vi "Q14070-Z060B手动版.vi"() -> ()   [LabVIEW 2013]
uses:
  <vilib>/Utility/file.llb/Read From Spreadsheet File (string).vi
  <vilib>/express/express arith-compare/Formula/XNode/ExpressFormulaBlockNode.xnode
  PCI8622_32.dll
  <vilib>/printing/EasyPrintingControls.llb/contents.ctl
  <vilib>/Utility/NIReport.llb/NI_ReportGenerationCore.lvlib
  <vilib>/printing/EasyPrintingControls.llb/report_type.ctl
  <vilib>/Utility/NIReport.llb/NI_report.lvclass
  <vilib>/printing/EasyPrinting.llb/Easy Print VI Panel or Documentation (path).vi
panel:
  out "界面启动":bool
  out "间隙扭矩扳手信号":bool
  out "齿条右极限":dbl
  out "齿条左极限":dbl
  out "左轴向力数组大小":i32
  in  "电动缸快速":dbl=10.0
  in  "电动缸慢速":dbl=1.0
  out "最大轴向力标准(N)":dbl=200.0 caption="L+Lmax(mm)" format="%#.3f"
  out "循环退出":bool
  in  "?":bool
  in  "密码":string
  in  "?":bool
  in  "?":bool
  in  "截取百分比":dbl=0.05
  in  "半行程":dbl=70.0
  out "PLC":bool
  out "齿条传动比":dbl=200.0 caption="L+Lmax(mm)" format="%#.3f"
  out "右平均轴向力(N)":dbl caption="L+Lmax(mm)" format="%#.3f"
  out "左平均轴向力(N)":dbl caption="最大位移偏离Lmax(mm)" format="%#.3f"
  in  "确定按钮":bool
  out "员工ID":string
  in  "出支线工步号":dbl
  out "报警提示":string
  in  "报警工步号":dbl
  out "急停":bool
  out "DeviceHandle":u32
  in  "轴向力设定次数":dbl=5.0
  in  "最小间隙(mm)":dbl=0.0005 format="%#.3f"
  out "本备料状态H":bool
  out "本测试状态H":bool
  out "本自动状态H":bool
  out "夹头松开":bool
  out "测头右位":bool
  out "测头左位":bool
  in  "测头气缸右移":bool
  in  "测头气缸左移":bool
  in  "轴向力已做次数":dbl
  out "轴向力及全行程间隙合格":bool
  out "轴向力启动":bool
  out "间隙启动":bool
  out "夹头夹紧位":bool
  in  "夹头松开":bool
  in  "夹头夹紧":bool
  out "error out":errorcluster
  out "型号数量":i32
  out "error out 4":errorcluster
  in  "间隙设定调整次数":dbl=5.0
  out "读取产品ID":string
  out "本备料状态":bool
  out "本测试状态":bool
  out "本自动状态":bool
  out "FGCS":string
  out "KSJJ":string
  out "Z060BRFID":string
  out "轴向力Y":dbl[](array[numeric])
  out "轴向力X":dbl[](array[numeric])
  out "间隙X数组":dbl[](array[numeric])
  out "间隙Y数组":dbl[](array[numeric])
  out "error out 3":errorcluster caption="错误输出"
  out "rfid工步号":u32
  out "芯片ID":string="201209190001"
  out "rfid完成":bool
  out "rfid触发":bool
  out "本序已做":bool
  in  "回零完成":bool
  in  "电动缸回零":bool
  in  "单点间隙已调试次数":dbl
  in  "需调整角度(度)":dbl
  in  "转向器中心":dbl
  out "扭矩到达":bool
  out "黄灯":bool
  out "红灯":bool
  out "基准位移":dbl caption="压力传感器" format="%#.4f"
  out "上序不合格":bool
  out "单点间隙合格":bool
  out "上序合格":bool
  out "测头机构电机":u32
  out "复位":bool
  in  "型号选择":u16(ring)=2 items=["J709", "J728", "J706"]
  in  "联线按钮":bool
  in  "工步号":u32
  in  "产品ID":string="201209190001"
  out "间隙位移(mm)":dbl=-4.6787895475327215 caption="压力传感器" format="%#.3f"
  out "齿条推拉力(N)":dbl format="%#.2f"
  out "齿条扭矩(Nm)":dbl format="%#.2f"
  out "通讯状态":bool
  out "员工姓名":string
  out "工步提示":string
  out "ADODB._Connection Out 2":refnum<k7>
  out "旋转齿条电机":u32
  out "电动缸电机":u32
  in  "停止":bool
  in  "参数加载":bool
  in  "选项卡控件":T1(tab)
  out "180°外全行程间隙标准(mm)":dbl=0.1 format="%#.3f"
  out "扭动曲线":cluster{"Y":dbl[], "Y":dbl[]}[](graph) caption="压球涨堵头1"
  out "中间位置间隙":dbl caption="间隙值L(mm)" format="%#.3f"
  in  "中间位置最大间隙标准(mm)":dbl=0.07 format="%#.3f"
  out "右180°外全行程间隙":dbl caption="正向最大间隙L1(mm)" format="%#.3f"
  out "左180°外全行程间隙":dbl caption="正向最大间隙L1(mm)" format="%#.3f"
  out "右180°内全行程间隙":dbl caption="正向最大间隙L1(mm)" format="%#.3f"
  out "左180°内全行程间隙":dbl caption="正向最大间隙L1(mm)" format="%#.3f"
  out "180°内全行程间隙标准(mm)":dbl=0.07 format="%#.3f"
  in  "找帽OK":bool
  out "左全行程间隙":dbl caption="正向最大间隙L1(mm)" format="%#.3f"
  out "右全行程间隙":dbl caption="正向最大间隙L1(mm)" format="%#.3f"
  out "总圈数最大值":dbl
  out "总圈数标准":dbl
  out "总行程最大值":dbl
  out "总行程标准(mm)":dbl
  out "力波动标准(N)":dbl=60.0 caption="L+Lmax(mm)" format="%#.3f"
  out "轴向力标准(N)":dbl=100.0 caption="L+Lmax(mm)" format="%#.3f"
  out "右轴向力波动(N)":dbl caption="L+Lmax(mm)" format="%_4g"
  out "右最大轴向力(N)":dbl caption="L+Lmax(mm)" format="%_4g"
  out "左轴向力波动(N)":dbl caption="最大位移偏离Lmax(mm)" format="%_4g"
  out "左最大轴向力(N)":dbl caption="最大位移偏离Lmax(mm)" format="%_4g"
  out "行程跳动曲线":cluster{"Y":dbl[], "Y":dbl[]}[](graph) caption="压球涨堵头1"
  out "平均轴向力标准(N) max":dbl=200.0 caption="L+Lmax(mm)" format="%#.3f"
  out "总行程":dbl format="%_4g"
  out "总圈数":dbl format="%_4g"
  in  "不合格品":bool
  in  "齿条右极限":dbl=-70.0 caption="压力传感器" format="%#.2f"
  in  "齿条左极限":dbl=-262.0 caption="压力传感器" format="%#.2f"
  in  "齿条移动速度":dbl=5.0 caption="压力传感器" format="%#.2f"
  in  "旋转齿条轴找帽转速":dbl=5.0 caption="压力传感器" format="%#.2f"
  in  "测量点扭矩":dbl=4.0 caption="压力传感器" format="%#.2f"
  in  "旋转齿条轴测量转速":dbl caption="压力传感器" format="%#.2f"
  in  "测头机构轴后退位":dbl=30.0 caption="压力传感器" format="%#.2f"
  in  "测头机构轴待检位":dbl caption="压力传感器" format="%#.2f"
  in  "测头机构轴检测位":dbl caption="压力传感器" format="%#.2f"
  in  "测头机构轴移动速度":dbl caption="压力传感器" format="%#.2f"
  in  "机械间隙值":dbl=3.5
  in  "阻挡":bool
  in  "放行":bool
  in  "夹头松开":bool
  in  "夹头夹紧":bool
  in  "测头气缸右移":bool
  in  "测头气缸左移":bool
  in  "支线下降":bool
  in  "支线顶升":bool
  in  "出支线":bool
  in  "进支线":bool
  in  "主线下降":bool
  in  "主线顶升":bool
  in  "下阻挡器放行":bool
  in  "上阻挡器放行":bool
  in  "测头机构轴使能":bool
  in  "测头机构轴后退":bool
  in  "测头机构轴前进":bool
  in  "电动缸速度(mm/s)":dbl=10.0 format="%#.3f"
  out "电动缸位置(mm)":dbl format="%#.3f"
  in  "旋转齿条轴速度(°/s)":dbl=10.0 format="%#.3f"
  out "旋转齿条轴位置(°)":dbl format="%#.3f"
  in  "测头机构轴速度(mm/s)":dbl=10.0 format="%#.3f"
  out "测头机构轴位置(mm)":dbl format="%#.3f"
  in  "旋转齿条轴右转":bool
  in  "旋转齿条轴左转":bool
  in  "旋转齿条轴使能":bool
  in  "电动缸后退":bool
  in  "电动缸使能":bool
  in  "电动缸前进":bool
  in  "齿条扭矩比例偏移":dbl=1.0 format="%#.2f"
  in  "齿条扭矩零点偏移":dbl format="%#.2f"
  in  "齿条推拉力比例偏移":dbl=1.0 format="%#.2f"
  in  "齿条推拉力零点偏移":dbl format="%#.2f"
  in  "间隙位移比例偏移":dbl=1.0 format="%#.2f"
  in  "间隙位移零点偏移":dbl format="%#.2f"
  in  "传感器参数保存":bool
  in  "参数修改":bool
  in  "参数查询":bool
  in  "参数浏览表":string[][](table)
  # "芜湖机械转向器装配线"
  # "间隙及轴向力检测"
  # "湖北唯思凌科装备制造有限公司 设计开发 (C)2015"
  # "Q14070机械转向器装配线"
  # "≤"
  # "间隙测量结果"
  # "间隙测量判定值"
  # "≤"
  # "≤"
  # "≤"
  # "轴向力测量结果"
  # "轴向力测量标准"
  # "≥"
  # "≤"
  # "≥"
  # "≤"
  # "≤"
  # "≥"
  # "不得大于20NM"
  # "传感器校验区"
  # "关于传感器校验：\n1、传感器校验需要由具备资质的单位或部门进行校验。\n2、具备权限的用户才能够修改传感器校验参数和试验参数。\n3、修改校验参数方法：先将比例偏移置为1，修改零点偏移，使零点值与校验的传感器一致；然后根据增幅调整比例偏移。"
  # "注意：\n具备权限的用户才能够修改传感器校验参数和试验参数！"
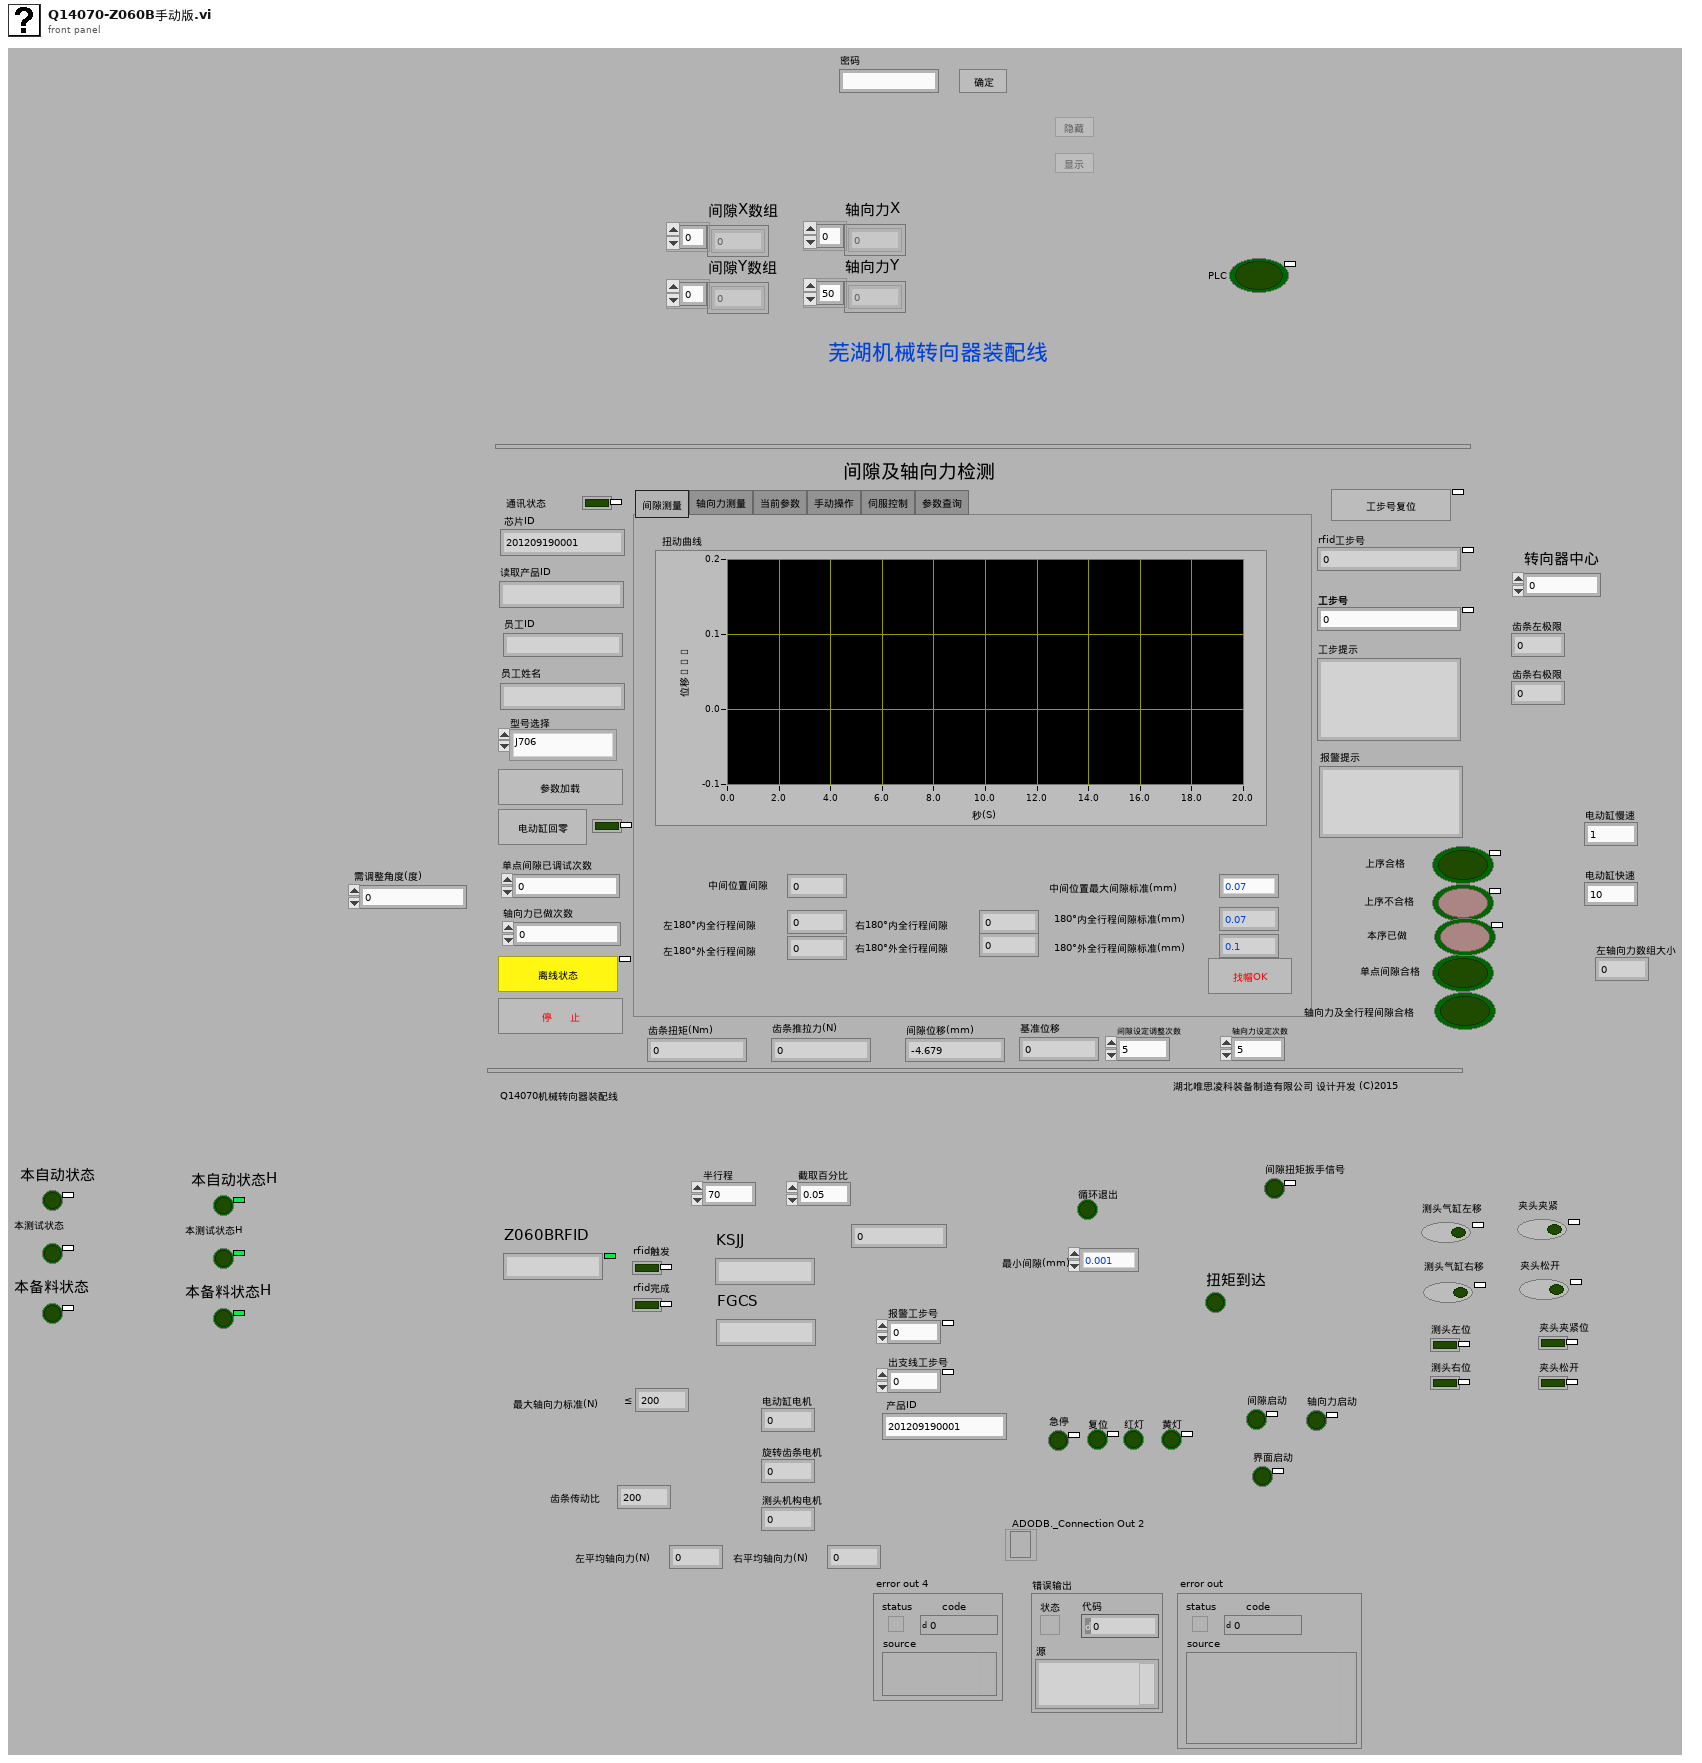
[diagram p1: front panel]
types:
  T1 = enum32{"间隙测量", "轴向力测量", "当前参数", "手动操作", "伺服控制", "传感器校验", "参数查询"}
  T2 = typedef "NI_ReportGenerationCore.lvlib/report_type.ctl" = u16
  T3 = typedef "NI_ReportGenerationCore.lvlib/contents.ctl" = u16
  T4 = typedef "imagedata.ctl" = cluster{"image type":i32, "image depth":i32, "image":u8[], "mask":u8[], "colors":u32[], "Rectangle":cluster{"left":i16, "top":i16, "right":i16, "bottom":i16}}
  T5 = enum8{"Enabled", "Disabled", "Disabled and Grayed Out"}
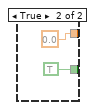
[diagram p2: hidden frame]
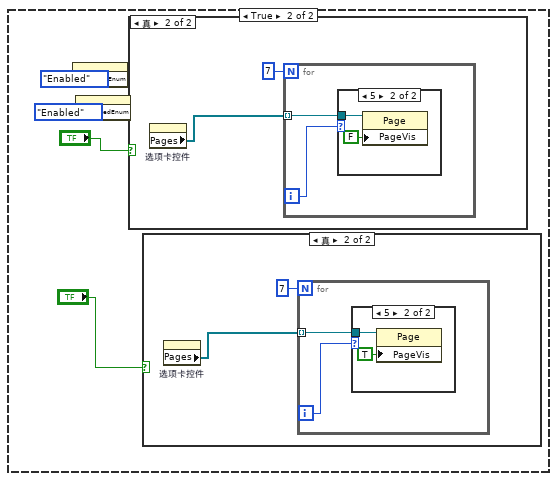
[diagram p4: hidden frame]
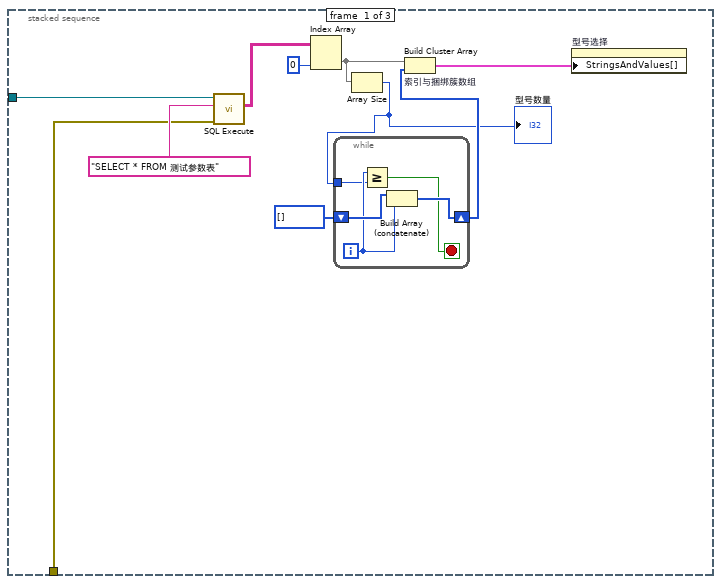
[diagram p11: hidden frame]
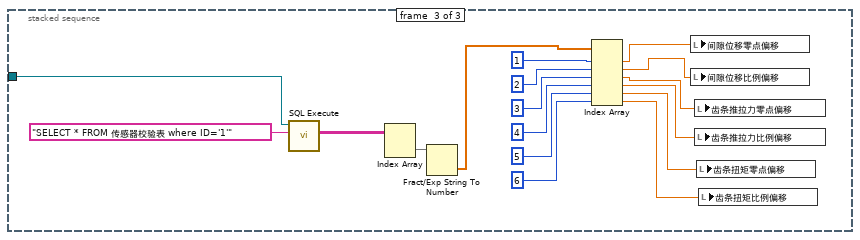
[diagram p12: hidden frame]
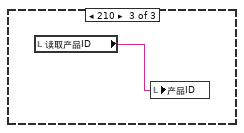
[diagram p14: hidden frame]
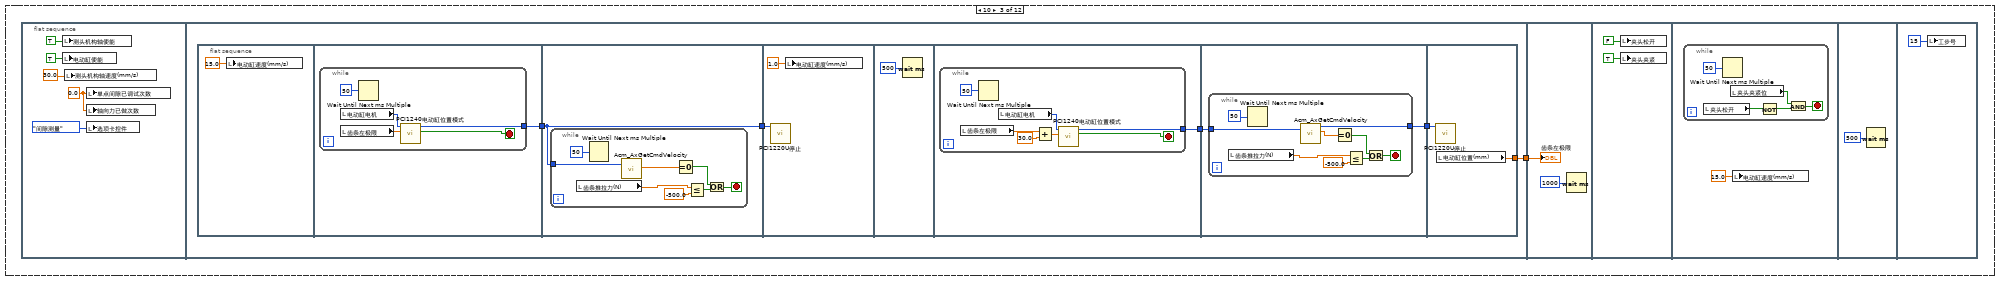
[diagram p17: hidden frame]
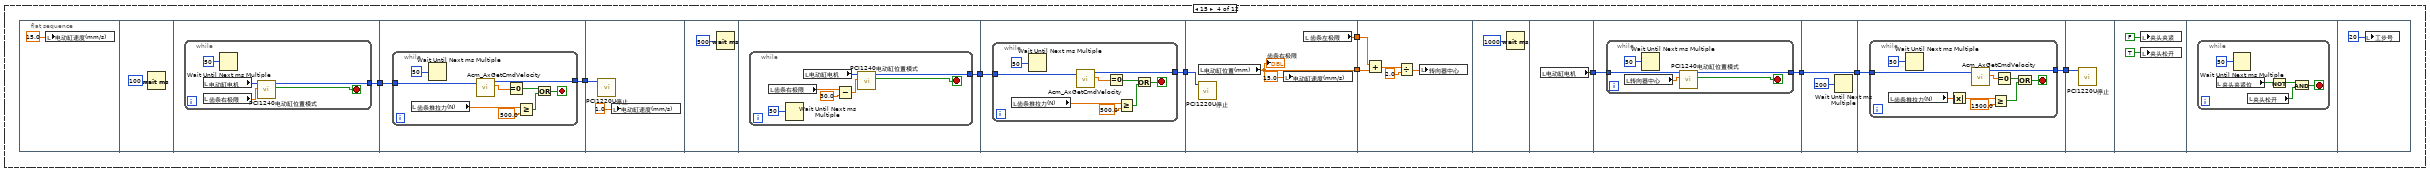
[diagram p18: hidden frame]
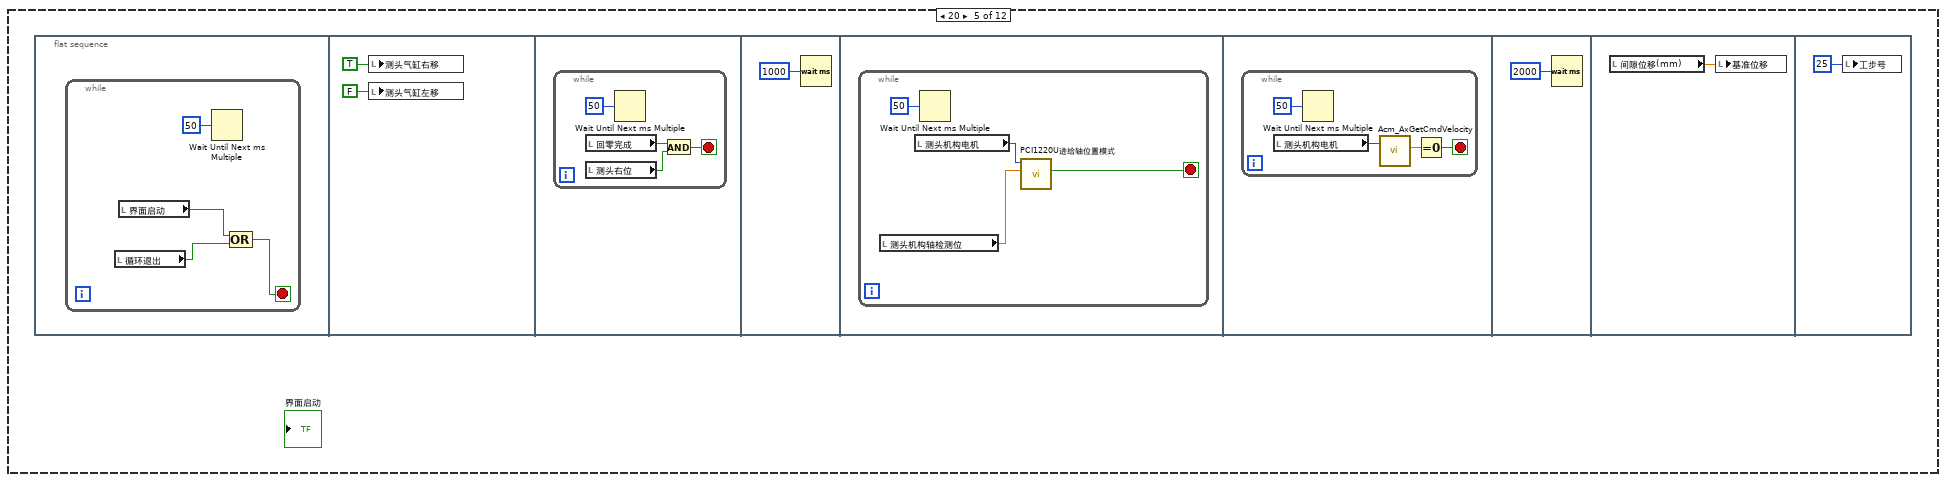
[diagram p19: hidden frame]
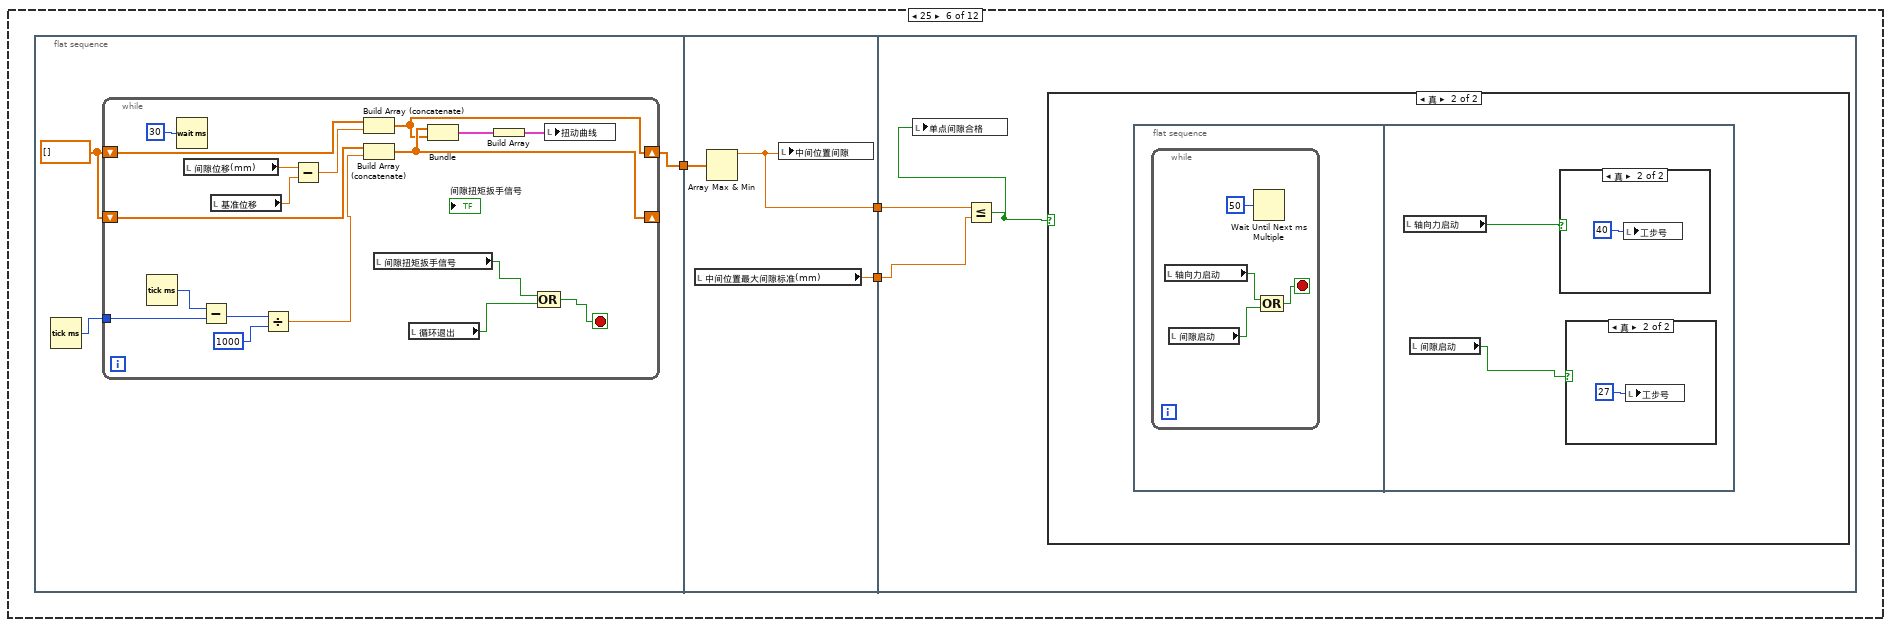
[diagram p20: hidden frame]
diagram:
  n1 = while {
    stop <- w7 stop-if-true
    n2 = local read "工步号"() -> (w5:u32)
    n3 = case shown="40" w5 {
      frame 0, Default {
      }
      frame 6 {
      }
      frame 10 {
        n4 = flat-sequence {
          tunnel: [w17] -> w8
          tunnel: w8 -> [w59]
          frame #0 {
            w9 = 0.0 ("已调试次数")
            n5 = local write "测头机构轴使能"(TRUE ("调整机构轴使能")) -> ()
            n6 = local write "电动缸使能"(TRUE ("电动缸使能")) -> ()
            n7 = local write "测头机构轴速度(mm/s)"(30.0 ("调整机构轴速度(mm/s)")) -> ()
            n8 = local write "单点间隙已调试次数"(w9) -> ()
            n9 = local write "轴向力已做次数"(w9) -> ()
            n10 = local write "选项卡控件"(T1."间隙测量" ("选项卡控件")) -> ()
          }
          frame #1 {
            n11 = flat-sequence {
              tunnel: [w20] -> w18
              tunnel: w18 -> [w26]
              tunnel: [w26] -> w16
              tunnel: w16 -> [w36]
              tunnel: [w38] -> w15
              tunnel: w15 -> [w47]
              tunnel: [w46] -> w14
              tunnel: [w58] -> w17
              tunnel: w14 -> [w57]
              frame #0 {
                n12 = local write "电动缸速度(mm/s)"(15.0 ("电动缸速度(mm/s)")) -> ()
              }
              frame #1 {
                n13 = while {
                  tunnel: [w24] -> w20
                  stop <- w23 stop-if-true
                  n14 = local read "电动缸电机"() -> (w25:u32)
                  n15 = local read "齿条左极限"() -> (w21:dbl)
                  n16 = Wait Until Next ms Multiple(millisecond multiple=u32 50 ("毫秒倍数")) -> ()  [unwired: 1 out]
                  n17 = call "PCI1240电动缸位置模式 .vi"("Distance"=w21, "AxisHandle IN"=w25) -> ("AbsSuccess"=w23:bool, "AxisHandle OUT"=w24:u32)  [unwired: 8 in]
                }
              }
              frame #2 {
                n18 = while {
                  tunnel: w26 -> [w33]
                  stop <- w30 stop-if-true
                  n19 = local read "齿条推拉力(N)"() -> (w27:dbl)
                  n20 = Wait Until Next ms Multiple(millisecond multiple=u32 50 ("毫秒倍数")) -> ()  [unwired: 1 out]
                  n21 = call <userlib>:"Acm_AxGetCmdVelocity.vi"("AxisHandle"=w33) -> ("Velocity"=w34:dbl)  [unwired: 1 in, 3 out]
                  n22 = Equal To 0?(x=w34) -> (x = 0?=w31:bool)
                  n23 = Less Or Equal?(x=w27, y=-500.0) -> (x <= y?=w28:bool)
                  n24 = Or(x=w31, y=w28) -> (x .or. y?=w30:bool)
                }
              }
              frame #3 {
                n25 = call "PCI1220U停止.vi"("AxisHandle IN"=w36) -> ()  [unwired: 9 in, 2 out]
                n26 = local write "电动缸速度(mm/s)"(1.0 ("电动缸速度(mm/s)")) -> ()
              }
              frame #4 {
                n27 = Wait (ms)(milliseconds to wait=u32 500 ("等待时间（毫秒）")) -> ()  [unwired: 1 out]
              }
              frame #5 {
                n28 = while {
                  tunnel: [w44] -> w38
                  stop <- w43 stop-if-true
                  n29 = local read "齿条左极限"() -> (w40:dbl)
                  n30 = Wait Until Next ms Multiple(millisecond multiple=u32 50 ("毫秒倍数")) -> ()  [unwired: 1 out]
                  n31 = local read "电动缸电机"() -> (w45:u32)
                  n32 = Add(x=w40, y=30.0) -> (x+y=w41:dbl)
                  n33 = call "PCI1240电动缸位置模式 .vi"("Distance"=w41, "AxisHandle IN"=w45) -> ("AbsSuccess"=w43:bool, "AxisHandle OUT"=w44:u32)  [unwired: 8 in]
                }
              }
              frame #6 {
                n34 = while {
                  tunnel: w47 -> [w55]
                  tunnel: [w49] -> w46
                  stop <- w52 stop-if-true
                  n35 = local read "齿条推拉力(N)"() -> (w48:dbl)
                  n36 = Wait Until Next ms Multiple(millisecond multiple=u32 50 ("毫秒倍数")) -> ()  [unwired: 1 out]
                  n37 = call <userlib>:"Acm_AxGetCmdVelocity.vi"("AxisHandle"=w55) -> ("Velocity"=w56:dbl, "AxisHandle"=w49:u32)  [unwired: 1 in, 2 out]
                  n38 = Equal To 0?(x=w56) -> (x = 0?=w53:bool)
                  n39 = Less Or Equal?(x=w48, y=-500.0) -> (x <= y?=w50:bool)
                  n40 = Or(x=w53, y=w50) -> (x .or. y?=w52:bool)
                }
              }
              frame #7 {
                n41 = call "PCI1220U停止.vi"("AxisHandle IN"=w57) -> ()  [unwired: 9 in, 2 out]
                n42 = local read "电动缸位置(mm)"() -> (w58:dbl)
              }
            }
          }
          frame #2 {
            n43 = Wait (ms)(milliseconds to wait=u32 1000 ("毫秒倍数")) -> ()  [unwired: 1 out]
            "齿条左极限" <- w59
          }
          frame #3 {
            n44 = local write "夹头松开"(FALSE ("夹头松开")) -> ()
            n45 = local write "夹头夹紧"(TRUE ("夹头夹紧")) -> ()
          }
          frame #4 {
            n46 = while {
              stop <- w65 stop-if-true
              n47 = local read "夹头松开"() -> (w68:bool)
              n48 = Wait Until Next ms Multiple(millisecond multiple=u32 50 ("毫秒倍数")) -> ()  [unwired: 1 out]
              n49 = local read "夹头夹紧位"() -> (w66:bool)
              n50 = Not(x=w68) -> (.not. x?=w67:bool)
              n51 = And(x=w66, y=w67) -> (x .and. y?=w65:bool)
            }
            n52 = local write "电动缸速度(mm/s)"(15.0 ("电动缸速度(mm/s)")) -> ()
          }
          frame #5 {
            n53 = Wait (ms)(milliseconds to wait=u32 500 ("等待时间（毫秒）")) -> ()  [unwired: 1 out]
          }
          frame #6 {
            n54 = local write "工步号"(u32 15 ("工步号")) -> ()
          }
        }
      }
      frame 15 {
        n55 = flat-sequence {
          tunnel: [w83] -> w80
          tunnel: w80 -> [w90]
          tunnel: [w89] -> w79
          tunnel: w79 -> [w101]
          tunnel: [w103] -> w78
          tunnel: w78 -> [w112]
          tunnel: [w111] -> w77
          tunnel: [w125] -> w76
          tunnel: [w124] -> w75
          tunnel: w77 -> [w123]
          tunnel: w76 -> [w130]
          tunnel: w75 -> [w129]
          tunnel: [w132] -> w74
          tunnel: [w134] -> w73
          tunnel: w74 -> [w133]
          tunnel: [w140] -> w72
          tunnel: w73 -> [w140]
          tunnel: w72 -> [w143]
          tunnel: [w142] -> w71
          tunnel: w71 -> [w154]
          frame #0 {
            n56 = local write "电动缸速度(mm/s)"(15.0 ("电动缸速度(mm/s)")) -> ()
          }
          frame #1 {
            n57 = Wait (ms)(milliseconds to wait=u32 100 ("等待时间（毫秒）")) -> ()  [unwired: 1 out]
          }
          frame #2 {
            n58 = while {
              tunnel: [w86] -> w83
              stop <- w88 stop-if-true
              n59 = local read "电动缸电机"() -> (w85:u32)
              n60 = local read "齿条右极限"() -> (w84:dbl)
              n61 = Wait Until Next ms Multiple(millisecond multiple=u32 50 ("毫秒倍数")) -> ()  [unwired: 1 out]
              n62 = call "PCI1240电动缸位置模式 .vi"("Distance"=w84, "AxisHandle IN"=w85) -> ("AbsSuccess"=w88:bool, "AxisHandle OUT"=w86:u32)  [unwired: 8 in]
            }
          }
          frame #3 {
            n63 = while {
              tunnel: w90 -> [w99]
              tunnel: [w92] -> w89
              stop <- w93 stop-if-true
              n64 = local read "齿条推拉力(N)"() -> (w91:dbl)
              n65 = Wait Until Next ms Multiple(millisecond multiple=u32 50 ("毫秒倍数")) -> ()  [unwired: 1 out]
              n66 = call <userlib>:"Acm_AxGetCmdVelocity.vi"("AxisHandle"=w99) -> ("Velocity"=w98:dbl, "AxisHandle"=w92:u32)  [unwired: 1 in, 2 out]
              n67 = Equal To 0?(x=w98) -> (x = 0?=w95:bool)
              n68 = Greater Or Equal?(x=w91, y=500.0) -> (x >= y?=w94:bool)
              n69 = Or(x=w95, y=w94) -> (x .or. y?=w93:bool)
            }
          }
          frame #4 {
            n70 = call "PCI1220U停止.vi"("AxisHandle IN"=w101) -> ()  [unwired: 9 in, 2 out]
            n71 = local write "电动缸速度(mm/s)"(1.0 ("电动缸速度(mm/s)")) -> ()
          }
          frame #5 {
            n72 = Wait (ms)(milliseconds to wait=u32 500 ("等待时间（毫秒）")) -> ()  [unwired: 1 out]
          }
          frame #6 {
            n73 = while {
              tunnel: [w108] -> w103
              stop <- w110 stop-if-true
              n74 = local read "齿条右极限"() -> (w106:dbl)
              n75 = Wait Until Next ms Multiple(millisecond multiple=u32 50 ("毫秒倍数")) -> ()  [unwired: 1 out]
              n76 = local read "电动缸电机"() -> (w107:u32)
              n77 = Subtract(x=w106, y=30.0) -> (x-y=w105:dbl)
              n78 = call "PCI1240电动缸位置模式 .vi"("Distance"=w105, "AxisHandle IN"=w107) -> ("AbsSuccess"=w110:bool, "AxisHandle OUT"=w108:u32)  [unwired: 8 in]
            }
          }
          frame #7 {
            n79 = while {
              tunnel: w112 -> [w121]
              tunnel: [w114] -> w111
              stop <- w115 stop-if-true
              n80 = local read "齿条推拉力(N)"() -> (w113:dbl)
              n81 = Wait Until Next ms Multiple(millisecond multiple=u32 50 ("毫秒倍数")) -> ()  [unwired: 1 out]
              n82 = call <userlib>:"Acm_AxGetCmdVelocity.vi"("AxisHandle"=w121) -> ("Velocity"=w120:dbl, "AxisHandle"=w114:u32)  [unwired: 1 in, 2 out]
              n83 = Equal To 0?(x=w120) -> (x = 0?=w117:bool)
              n84 = Greater Or Equal?(x=w113, y=500.0) -> (x >= y?=w116:bool)
              n85 = Or(x=w117, y=w116) -> (x .or. y?=w115:bool)
            }
          }
          frame #8 {
            n86 = local read "电动缸位置(mm)"() -> (w124:dbl)
            "齿条右极限" <- w124
            n87 = call "PCI1220U停止.vi"("AxisHandle IN"=w123) -> ()  [unwired: 9 in, 2 out]
            n88 = local write "电动缸速度(mm/s)"(15.0 ("电动缸速度(mm/s)")) -> ()
            n89 = local read "齿条左极限"() -> (w125:dbl)
          }
          frame #9 {
            n90 = Add(x=w130, y=w129) -> (x+y=w128:dbl)
            n91 = Divide(x=w128, y=2.0) -> (x/y=w127:dbl)
            n92 = local write "转向器中心"(w127) -> ()
          }
          frame #10 {
            n93 = Wait (ms)(milliseconds to wait=u32 1000 ("等待时间（毫秒）")) -> ()  [unwired: 1 out]
          }
          frame #11 {
            n94 = local read "电动缸电机"() -> (w132:u32)
          }
          frame #12 {
            n95 = while {
              tunnel: w133 -> [w139]
              tunnel: [w136] -> w134
              stop <- w138 stop-if-true
              n96 = local read "转向器中心"() -> (w135:dbl)
              n97 = Wait Until Next ms Multiple(millisecond multiple=u32 50 ("毫秒倍数")) -> ()  [unwired: 1 out]
              n98 = call "PCI1240电动缸位置模式 .vi"("Distance"=w135, "AxisHandle IN"=w139) -> ("AbsSuccess"=w138:bool, "AxisHandle OUT"=w136:u32)  [unwired: 8 in]
            }
          }
          frame #13 {
            n99 = Wait Until Next ms Multiple(millisecond multiple=u32 200 ("毫秒倍数")) -> ()  [unwired: 1 out]
          }
          frame #14 {
            n100 = while {
              tunnel: w143 -> [w153]
              tunnel: [w144] -> w142
              stop <- w145 stop-if-true
              n101 = local read "齿条推拉力(N)"() -> (w150:dbl)
              n102 = Wait Until Next ms Multiple(millisecond multiple=u32 50 ("毫秒倍数")) -> ()  [unwired: 1 out]
              n103 = Absolute Value(x=w150) -> (abs(x)=w149:dbl)
              n104 = call <userlib>:"Acm_AxGetCmdVelocity.vi"("AxisHandle"=w153) -> ("Velocity"=w152:dbl, "AxisHandle"=w144:u32)  [unwired: 1 in, 2 out]
              n105 = Greater Or Equal?(x=w149, y=1500.0) -> (x >= y?=w146:bool)
              n106 = Equal To 0?(x=w152) -> (x = 0?=w147:bool)
              n107 = Or(x=w147, y=w146) -> (x .or. y?=w145:bool)
            }
          }
          frame #15 {
            n108 = call "PCI1220U停止.vi"("AxisHandle IN"=w154) -> ()  [unwired: 9 in, 2 out]
          }
          frame #16 {
            n109 = local write "夹头夹紧"(FALSE ("夹头夹紧")) -> ()
            n110 = local write "夹头松开"(TRUE ("夹头松开")) -> ()
          }
          frame #17 {
            n111 = while {
              stop <- w160 stop-if-true
              n112 = local read "夹头夹紧位"() -> (w161:bool)
              n113 = Wait Until Next ms Multiple(millisecond multiple=u32 50 ("毫秒倍数")) -> ()  [unwired: 1 out]
              n114 = local read "夹头松开"() -> (w157:bool)
              n115 = Not(x=w161) -> (.not. x?=w158:bool)
              n116 = And(x=w158, y=w157) -> (x .and. y?=w160:bool)
            }
          }
          frame #18 {
            n117 = local write "工步号"(u32 20 ("工步号")) -> ()
          }
        }
      }
      frame 20 {
        n118 = flat-sequence {
          frame #0 {
            n119 = while {
              stop <- w164 stop-if-true
              n120 = local read "循环退出"() -> (w166:bool)
              n121 = local read "界面启动"() -> (w165:bool)
              n122 = Wait Until Next ms Multiple(millisecond multiple=u32 50 ("毫秒倍数")) -> ()  [unwired: 1 out]
              n123 = Compound Arithmetic op=OR(w165, w166) -> (w164:bool)
            }
          }
          frame #1 {
            n124 = local write "测头气缸右移"(TRUE ("测头气缸右移")) -> ()
            n125 = local write "测头气缸左移"(FALSE ("测头气缸左移")) -> ()
          }
          frame #2 {
            n126 = while {
              stop <- w169 stop-if-true
              n127 = local read "回零完成"() -> (w171:bool)
              n128 = local read "测头右位"() -> (w170:bool)
              n129 = Wait Until Next ms Multiple(millisecond multiple=u32 50 ("毫秒倍数")) -> ()  [unwired: 1 out]
              n130 = And(x=w171, y=w170) -> (x .and. y?=w169:bool)
            }
          }
          frame #3 {
            n131 = Wait (ms)(milliseconds to wait=u32 1000 ("等待时间（毫秒）")) -> ()  [unwired: 1 out]
          }
          frame #4 {
            n132 = while {
              stop <- w177 stop-if-true
              n133 = local read "测头机构轴检测位"() -> (w174:dbl)
              n134 = local read "测头机构电机"() -> (w175:u32)
              n135 = Wait Until Next ms Multiple(millisecond multiple=u32 50 ("毫秒倍数")) -> ()  [unwired: 1 out]
              n136 = call "PCI1220U进给轴位置模式.vi"("Distance"=w174, "AxisHandle IN"=w175) -> ("AbsSuccess"=w177:bool)  [unwired: 8 in, 1 out]
            }
          }
          frame #5 {
            n137 = while {
              stop <- w180 stop-if-true
              n138 = local read "测头机构电机"() -> (w178:u32)
              n139 = Wait Until Next ms Multiple(millisecond multiple=u32 50 ("毫秒倍数")) -> ()  [unwired: 1 out]
              n140 = call <userlib>:"Acm_AxGetCmdVelocity.vi"("AxisHandle"=w178) -> ("Velocity"=w181:dbl)  [unwired: 1 in, 3 out]
              n141 = Equal To 0?(x=w181) -> (x = 0?=w180:bool)
            }
          }
          frame #6 {
            n142 = Wait (ms)(milliseconds to wait=u32 2000 ("等待时间（毫秒）")) -> ()  [unwired: 1 out]
          }
          frame #7 {
            n143 = local read "间隙位移(mm)"() -> (w183:dbl)
            n144 = local write "基准位移"(w183) -> ()
          }
          frame #8 {
            n145 = local write "工步号"(u32 25 ("工步号")) -> ()
          }
        }
      }
      frame 25 {
        n146 = flat-sequence {
          tunnel: [w188] -> w187
          tunnel: w187 -> [w211]
          tunnel: [w210] -> w186
          tunnel: [w209] -> w185
          tunnel: w186 -> [w214]
          tunnel: w185 -> [w213]
          frame #0 {
            w190 = dbl[] []
            n147 = Tick Count (ms)() -> (millisecond timer value=w189:u32)
            n148 = while {
              shift-right: [w205] -> _
              shift-left: w190 -> [w207]
              shift-right: [w204] -> w188
              shift-left: w190 -> [w206]
              tunnel: w189 -> [w197]
              stop <- w193 stop-if-true
              n149 = Tick Count (ms)() -> (millisecond timer value=w198:u32)
              n150 = Wait (ms)(milliseconds to wait=u32 30 ("毫秒倍数")) -> ()  [unwired: 1 out]
              n151 = local read "间隙位移(mm)"() -> (w201:dbl)
              n152 = Subtract(x=w198, y=w197) -> (x-y=w196:u32)
              n153 = local read "基准位移"() -> (w199:dbl)
              n154 = Divide(x=w196, y=u32 1000) -> (x/y=w194:dbl)
              n155 = Subtract(x=w201, y=w199) -> (x-y=w200:dbl)
              n156 = Build Array (concatenate) ("创建数组")(w206, w200) -> (w204:dbl[])
              n157 = Build Array (concatenate) ("创建数组")(w207, w194) -> (w205:dbl[])
              n158 = local read "间隙扭矩扳手信号"() -> (w191:bool)
              n159 = local read "循环退出"() -> (w192:bool)
              n160 = Bundle ("捆绑")(w205, w204) -> (w202:cluster{dbl[], dbl[]})  [unwired: 1 in]
              n161 = Build Array ("创建数组")(w202) -> (w203:cluster{dbl[], dbl[]}[])
              n162 = Compound Arithmetic op=OR(w191, w192) -> (w193:bool)
              n163 = local write "扭动曲线"(w203) -> ()
            }
          }
          frame #1 {
            n164 = local read "中间位置最大间隙标准(mm)"() -> (w209:dbl)
            n165 = Array Max & Min(array=w211) -> (max value=w210:dbl)  [unwired: 3 out]
            n166 = local write "中间位置间隙"(w210) -> ()
          }
          frame #2 {
            n167 = Less Or Equal?(x=w214, y=w213) -> (x <= y?=w212:bool)
            n168 = local write "单点间隙合格"(w212) -> ()
            n169 = case shown="真" w212 {
              frame False {
                n170 = local read "单点间隙已调试次数"() -> (w217:dbl)
                n171 = Less?(x=w217, y="间隙设定调整次数") -> (x < y?=w216:bool)
                n172 = case shown="真" w216 {
                  frame False {
                    n173 = local write "工步号"(u32 45 ("变更工步号")) -> ()
                  }
                  frame True {
                    n174 = local write "工步号"(u32 27 ("工步号")) -> ()
                  }
                }
              }
              frame True {
                n175 = flat-sequence {
                  frame #0 {
                    n176 = while {
                      stop <- w222 stop-if-true
                      n177 = local read "轴向力启动"() -> (w221:bool)
                      n178 = local read "间隙启动"() -> (w220:bool)
                      n179 = Wait Until Next ms Multiple(millisecond multiple=u32 50 ("毫秒倍数")) -> ()  [unwired: 1 out]
                      n180 = Compound Arithmetic op=OR(w221, w220) -> (w222:bool)
                    }
                  }
                  frame #1 {
                    n181 = local read "轴向力启动"() -> (w225:bool)
                    n182 = local read "间隙启动"() -> (w224:bool)
                    n183 = case shown="真" w225 {
                      frame False {
                      }
                      frame True {
                        n184 = local write "工步号"(u32 40 ("工步号")) -> ()
                      }
                    }
                    n185 = case shown="真" w224 {
                      frame False {
                      }
                      frame True {
                        n186 = local write "工步号"(u32 27 ("工步号")) -> ()
                      }
                    }
                  }
                }
              }
            }
          }
        }
      }
      frame 27 {
        n187 = flat-sequence {
          frame #0 {
            n188 = local read "单点间隙已调试次数"() -> (w230:dbl)
            n189 = Wait (ms)(milliseconds to wait=u32 1000 ("等待时间（毫秒）")) -> ()  [unwired: 1 out]
            n190 = Add(x=w230, y=1.0 ("已调试次数")) -> (x+y=w228:dbl)
            n191 = local write "单点间隙已调试次数"(w228) -> ()
          }
          frame #1 {
            n192 = while {
              stop <- w235 stop-if-true
              n193 = local read "测头机构轴后退位"() -> (w232:dbl)
              n194 = local read "测头机构电机"() -> (w233:u32)
              n195 = Wait Until Next ms Multiple(millisecond multiple=u32 50 ("毫秒倍数")) -> ()  [unwired: 1 out]
              n196 = call "PCI1220U进给轴位置模式.vi"("Distance"=w232, "AxisHandle IN"=w233) -> ("AbsSuccess"=w235:bool)  [unwired: 8 in, 1 out]
            }
          }
          frame #2 {
            n197 = while {
              stop <- w238 stop-if-true
              n198 = local read "测头机构电机"() -> (w236:u32)
              n199 = Wait Until Next ms Multiple(millisecond multiple=u32 50 ("毫秒倍数")) -> ()  [unwired: 1 out]
              n200 = call <userlib>:"Acm_AxGetCmdVelocity.vi"("AxisHandle"=w236) -> ("Velocity"=w239:dbl)  [unwired: 1 in, 3 out]
              n201 = Equal To 0?(x=w239) -> (x = 0?=w238:bool)
            }
          }
          frame #3 {
            n202 = Wait (ms)(milliseconds to wait=u32 2000 ("等待时间（毫秒）")) -> ()  [unwired: 1 out]
          }
          frame #4 {
            n203 = local write "测头气缸右移"(FALSE ("测头气缸右移")) -> ()
            n204 = local write "测头气缸左移"(TRUE ("测头气缸左移")) -> ()
          }
          frame #5 {
            n205 = local write "工步号"(u32 20 ("工步号")) -> ()
          }
        }
      }
      frame 30 {
        # "人工调整"
        n206 = flat-sequence {
          tunnel: [w246] -> w244
          tunnel: w244 -> [w253]
          frame #0 {
            n207 = local write "测头机构轴速度(mm/s)"(30.0 ("测头机构轴速度(mm/s)")) -> ()
          }
          frame #1 {
            n208 = local read "测头机构电机"() -> (w247:u32)
            n209 = while {
              tunnel: w247 -> [w250]
              tunnel: [w249] -> w246
              stop <- w252 stop-if-true
              n210 = local read "测头机构轴后退位"() -> (w248:dbl)
              n211 = call "PCI1220U进给轴位置模式.vi"("Distance"=w248, "AxisHandle IN"=w250) -> ("AbsSuccess"=w252:bool, "AxisHandle OUT"=w249:u32)  [unwired: 8 in]
              n212 = Wait Until Next ms Multiple(millisecond multiple=u32 50 ("毫秒倍数")) -> ()  [unwired: 1 out]
            }
          }
          frame #2 {
            n213 = while {
              tunnel: w253 -> [w257]
              stop <- w255 stop-if-true
              n214 = call <userlib>:"Acm_AxGetCmdVelocity.vi"("AxisHandle"=w257) -> ("Velocity"=w256:dbl)  [unwired: 1 in, 3 out]
              n215 = Wait Until Next ms Multiple(millisecond multiple=u32 50 ("毫秒倍数")) -> ()  [unwired: 1 out]
              n216 = Equal To 0?(x=w256) -> (x = 0?=w255:bool)
            }
          }
          frame #3 {
            n217 = while {
              stop <- w259 stop-if-true
              n218 = local read "测头机构轴位置(mm)"() -> (w261:dbl)
              n219 = Wait Until Next ms Multiple(millisecond multiple=u32 50 ("毫秒倍数")) -> ()  [unwired: 1 out]
              n220 = Less Or Equal?(x=w261, y=35.0) -> (x <= y?=w259:bool)
            }
          }
          frame #4 {
            n221 = local write "测头气缸左移"(TRUE ("测头气缸左移")) -> ()
            n222 = local write "测头气缸右移"(FALSE ("测头气缸右移")) -> ()
            n223 = local write "夹头松开"(TRUE ("测头气缸左移")) -> ()
            n224 = local write "夹头夹紧"(FALSE ("测头气缸右移")) -> ()
          }
          frame #5 {
            n225 = while {
              stop <- w266 stop-if-true
              # "等待启动"
              n226 = local read "间隙启动"() -> (w266:bool)
              n227 = Wait Until Next ms Multiple(millisecond multiple=u32 50 ("毫秒倍数")) -> ()  [unwired: 1 out]
            }
          }
          frame #6 {
            n228 = local read "不合格品"() -> (w268:bool)
            n229 = case shown="真" w268 {
              frame False {
                n230 = flat-sequence {
                  frame #0 {
                    n231 = local read "单点间隙已调试次数"() -> (w271:dbl)
                    n232 = local write "测头气缸左移"(FALSE ("测头气缸左移")) -> ()
                    n233 = local write "测头气缸右移"(TRUE ("测头气缸左移")) -> ()
                    n234 = Add(x=w271, y=1.0 ("已调试次数")) -> (x+y=w273:dbl)
                    n235 = local write "单点间隙已调试次数"(w273) -> ()
                  }
                  frame #1 {
                    n236 = while {
                      stop <- w274 stop-if-true
                      n237 = Wait Until Next ms Multiple(millisecond multiple=u32 50 ("毫秒倍数")) -> ()  [unwired: 1 out]
                      n238 = local read "测头右位"() -> (w274:bool)
                    }
                  }
                  frame #2 {
                    n239 = local write "工步号"(u32 20 ("工步号")) -> ()
                  }
                }
              }
              frame True {
                n240 = local write "工步号"(u32 45 ("工步号")) -> ()
              }
            }
          }
        }
      }
      frame 40 {
        n241 = flat-sequence {
          tunnel: [w401] -> w390
          tunnel: w390 -> [w403]
          tunnel: [w402] -> w389
          tunnel: w389 -> [w411]
          tunnel: [w411] -> w388
          tunnel: w388 -> [w423]
          tunnel: [w423] -> w387
          tunnel: w387 -> [w425]
          tunnel: [w424] -> w386
          tunnel: w386 -> [w433]
          tunnel: [w433] -> w385
          tunnel: w385 -> [w443]
          tunnel: [w443] -> w384
          tunnel: w384 -> [w451]
          tunnel: [w451] -> w383
          tunnel: w383 -> [w453]
          tunnel: [w454] -> w287
          tunnel: [w452] -> w286
          tunnel: w287 -> [w467]
          tunnel: w286 -> [w462]
          tunnel: [w465] -> w382
          tunnel: [w464] -> w381
          tunnel: [w463] -> w380
          tunnel: [w462] -> w379
          tunnel: [w504] -> w378
          tunnel: [w507] -> w377
          tunnel: w382 -> [w507]
          tunnel: [w506] -> w376
          tunnel: w381 -> [w506]
          tunnel: [w505] -> w375
          tunnel: w380 -> [w505]
          tunnel: w379 -> [w504]
          tunnel: w378 -> [w513]
          tunnel: [w509] -> w374
          tunnel: [w512] -> w373
          tunnel: w377 -> [w512]
          tunnel: [w511] -> w372
          tunnel: w376 -> [w511]
          tunnel: [w510] -> w371
          tunnel: w375 -> [w510]
          tunnel: [w508] -> w370
          tunnel: [w528] -> w366
          tunnel: [w527] -> w367
          tunnel: [w526] -> w368
          tunnel: w374 -> [w521]
          tunnel: w373 -> [w525]
          tunnel: w372 -> [w524]
          tunnel: w371 -> [w523]
          tunnel: w370 -> [w522]
          tunnel: [w521] -> w369
          tunnel: [w581] -> w285
          tunnel: [w566] -> w284
          tunnel: [w580] -> w283
          tunnel: [w579] -> w282
          tunnel: [w578] -> w281
          tunnel: [w577] -> w280
          tunnel: [w576] -> w279
          tunnel: w369 -> [w580]
          tunnel: w368 -> [w579]
          tunnel: w367 -> [w566]
          tunnel: w366 -> [w581]
          tunnel: [w567] -> w278
          tunnel: w285 -> [w603]
          tunnel: [w603] -> w365
          tunnel: w284 -> [w602]
          tunnel: [w602] -> w364
          tunnel: w283 -> [w601]
          tunnel: [w590] -> w363
          tunnel: [w589] -> w362
          tunnel: [w600] -> w361
          tunnel: w282 -> [w600]
          tunnel: w281 -> [w597]
          tunnel: w280 -> [w599]
          tunnel: w279 -> [w598]
          tunnel: [w592] -> w360
          tunnel: [w591] -> w359
          tunnel: w278 -> [w588]
          tunnel: w365 -> [w616]
          tunnel: w364 -> [w615]
          tunnel: w363 -> [w611]
          tunnel: w362 -> [w618]
          tunnel: [w618] -> w357
          tunnel: w361 -> [w617]
          tunnel: [w613] -> w356
          tunnel: w360 -> [w620]
          tunnel: [w620] -> w355
          tunnel: w359 -> [w619]
          tunnel: [w619] -> w354
          tunnel: [w614] -> w358
          tunnel: [w612] -> w353
          tunnel: [w611] -> w352
          tunnel: w358 -> [w665]
          tunnel: [w665] -> w351
          tunnel: [w659] -> w350
          tunnel: w357 -> [w664]
          tunnel: [w664] -> w349
          tunnel: w356 -> [w663]
          tunnel: [w663] -> w348
          tunnel: w355 -> [w662]
          tunnel: [w662] -> w347
          tunnel: w354 -> [w661]
          tunnel: [w661] -> w346
          tunnel: [w660] -> w345
          tunnel: w353 -> [w660]
          tunnel: w352 -> [w659]
          tunnel: w351 -> [w672]
          tunnel: [w672] -> w344
          tunnel: w350 -> [w666]
          tunnel: w349 -> [w671]
          tunnel: [w671] -> w343
          tunnel: w348 -> [w670]
          tunnel: [w670] -> w342
          tunnel: w347 -> [w669]
          tunnel: [w669] -> w341
          tunnel: w346 -> [w668]
          tunnel: [w668] -> w340
          tunnel: [w666] -> w339
          tunnel: [w667] -> w338
          tunnel: w345 -> [w667]
          tunnel: [w688] -> w337
          tunnel: [w687] -> w336
          tunnel: w344 -> [w680]
          tunnel: [w679] -> w335
          tunnel: w343 -> [w682]
          tunnel: [w682] -> w334
          tunnel: w342 -> [w683]
          tunnel: [w686] -> w333
          tunnel: w341 -> [w684]
          tunnel: w340 -> [w685]
          tunnel: [w685] -> w332
          tunnel: [w684] -> w331
          tunnel: w339 -> [w679]
          tunnel: w338 -> [w681]
          tunnel: w337 -> [w731]
          tunnel: w336 -> [w737]
          tunnel: [w737] -> w330
          tunnel: w335 -> [w734]
          tunnel: [w734] -> w329
          tunnel: w334 -> [w736]
          tunnel: [w736] -> w328
          tunnel: w333 -> [w735]
          tunnel: [w735] -> w327
          tunnel: [w731] -> w326
          tunnel: [w730] -> w325
          tunnel: [w729] -> w324
          tunnel: w332 -> [w727]
          tunnel: w331 -> [w728]
          tunnel: [w728] -> w323
          tunnel: [w727] -> w322
          tunnel: [w726] -> w321
          tunnel: w330 -> [w750]
          tunnel: [w784] -> w320
          tunnel: w329 -> [w784]
          tunnel: [w783] -> w319
          tunnel: w328 -> [w783]
          tunnel: w327 -> [w782]
          tunnel: [w780] -> w318
          tunnel: w326 -> [w779]
          tunnel: w325 -> [w777]
          tunnel: w324 -> [w776]
          tunnel: [w774] -> w317
          tunnel: [w773] -> w316
          tunnel: [w772] -> w315
          tunnel: [w747] -> w314
          tunnel: [w746] -> w313
          tunnel: w323 -> [w769]
          tunnel: w322 -> [w768]
          tunnel: [w769] -> w312
          tunnel: [w768] -> w311
          tunnel: [w767] -> w310
          tunnel: [w766] -> w309
          tunnel: [w763] -> w308
          tunnel: [w758] -> w307
          tunnel: [w753] -> w306
          tunnel: [w745] -> w305
          tunnel: w321 -> [w744]
          tunnel: w320 -> [w811]
          tunnel: [w811] -> w304
          tunnel: w319 -> [_]
          tunnel: [w808] -> w303
          tunnel: w318 -> [w810]
          tunnel: w317 -> [w806]
          tunnel: w316 -> [w805]
          tunnel: w315 -> [w804]
          tunnel: [w803] -> w302
          tunnel: [w802] -> w301
          tunnel: w314 -> [w801]
          tunnel: w313 -> [w800]
          tunnel: w312 -> [w796]
          tunnel: w311 -> [w795]
          tunnel: [w796] -> w300
          tunnel: [w795] -> w299
          tunnel: [w794] -> w298
          tunnel: [w793] -> w297
          tunnel: w310 -> [w793]
          tunnel: [w792] -> w296
          tunnel: w309 -> [w792]
          tunnel: [w791] -> w295
          tunnel: [w790] -> w294
          tunnel: w308 -> [w789]
          tunnel: [w788] -> w293
          tunnel: w307 -> [w788]
          tunnel: [w787] -> w292
          tunnel: w306 -> [w787]
          tunnel: w305 -> [w786]
          tunnel: w304 -> [w828]
          tunnel: [w828] -> w291
          tunnel: w303 -> [w827]
          tunnel: [w827] -> w290
          tunnel: w302 -> [w822]
          tunnel: w301 -> [w821]
          tunnel: w300 -> [w824]
          tunnel: w299 -> [w823]
          tunnel: w298 -> [w820]
          tunnel: w297 -> [w819]
          tunnel: w296 -> [w818]
          tunnel: w295 -> [w817]
          tunnel: w294 -> [w816]
          tunnel: w293 -> [w814]
          tunnel: w292 -> [w813]
          tunnel: w291 -> [w831]
          tunnel: [w830] -> w289
          tunnel: w290 -> [w829]
          tunnel: w289 -> [w838]
          tunnel: [w837] -> w288
          tunnel: w288 -> [w844]
          frame #0 {
            n242 = local write "夹头松开"(FALSE ("夹头松开")) -> ()
            n243 = local write "夹头夹紧"(TRUE ("夹头夹紧")) -> ()
          }
          frame #1 {
            n244 = while {
              stop <- w397 stop-if-true
              n245 = local read "夹头夹紧位"() -> (w394:bool)
              n246 = local read "夹头松开"() -> (w395:bool)
              n247 = Wait Until Next ms Multiple(millisecond multiple=u32 50 ("毫秒倍数")) -> ()  [unwired: 1 out]
              n248 = Not(x=w395) -> (.not. x?=w393:bool)
              n249 = And(x=w394, y=w393) -> (x .and. y?=w397:bool)
            }
          }
          frame #2 {
            n250 = local read "电动缸快速"() -> (w398:dbl)
            n251 = local write "电动缸速度(mm/s)"(w398) -> ()
            n252 = local write "单点间隙已调试次数"(0.0 ("单点间隙已调试次数")) -> ()
            n253 = local read "电动缸电机"() -> (w401:u32)
            n254 = local write "选项卡控件"(T1."轴向力测量" ("选项卡控件")) -> ()
          }
          frame #3 {
            n255 = while {
              tunnel: w403 -> [w410]
              tunnel: [w409] -> w402
              stop <- w404 stop-if-true
              n256 = local read "齿条左极限"() -> (w407:dbl)
              n257 = Wait (ms)(milliseconds to wait=u32 50 ("毫秒倍数")) -> ()  [unwired: 1 out]
              n258 = local read "循环退出"() -> (w406:bool)
              n259 = call "PCI1240电动缸位置模式 .vi"("Distance"=w407, "AxisHandle IN"=w410) -> ("AbsSuccess"=w405:bool, "AxisHandle OUT"=w409:u32)  [unwired: 8 in]
              n260 = Compound Arithmetic op=OR(w405, w406) -> (w404:bool)
            }
          }
          frame #4 {
            n261 = while {
              tunnel: w411 -> [w412]
              stop <- w414 stop-if-true
              n262 = local read "齿条推拉力(N)"() -> (w418:dbl)
              n263 = Wait (ms)(milliseconds to wait=u32 50 ("毫秒倍数")) -> ()  [unwired: 1 out]
              n264 = call <userlib>:"Acm_AxGetCmdVelocity.vi"("AxisHandle"=w412) -> ("Velocity"=w420:dbl)  [unwired: 1 in, 3 out]
              n265 = local read "循环退出"() -> (w413:bool)
              n266 = Less Or Equal?(x=w418, y=-500.0) -> (x <= y?=w415:bool)
              n267 = Equal To 0?(x=w420) -> (x = 0?=w416:bool)
              n268 = Compound Arithmetic op=OR(w416, w415, w413) -> (w414:bool)
            }
          }
          frame #5 {
            n269 = local read "电动缸慢速"() -> (w421:dbl)
            n270 = local write "电动缸速度(mm/s)"(w421) -> ()
            n271 = Wait (ms)(milliseconds to wait=u32 100 ("等待时间（毫秒）")) -> ()  [unwired: 1 out]
          }
          frame #6 {
            n272 = while {
              tunnel: w425 -> [w432]
              tunnel: [w430] -> w424
              stop <- w426 stop-if-true
              n273 = Wait (ms)(milliseconds to wait=u32 50 ("毫秒倍数")) -> ()  [unwired: 1 out]
              n274 = local read "循环退出"() -> (w428:bool)
              n275 = call "PCI1240电动缸位置模式 .vi"("Distance"=10000.0, "AxisHandle IN"=w432) -> ("AbsSuccess"=w427:bool, "AxisHandle OUT"=w430:u32)  [unwired: 8 in]
              n276 = Compound Arithmetic op=OR(w427, w428) -> (w426:bool)
            }
          }
          frame #7 {
            n277 = while {
              tunnel: w433 -> [w434]
              stop <- w436 stop-if-true
              n278 = local read "齿条推拉力(N)"() -> (w440:dbl)
              n279 = Wait (ms)(milliseconds to wait=u32 50 ("毫秒倍数")) -> ()  [unwired: 1 out]
              n280 = call <userlib>:"Acm_AxGetCmdVelocity.vi"("AxisHandle"=w434) -> ("Velocity"=w442:dbl)  [unwired: 1 in, 3 out]
              n281 = local read "循环退出"() -> (w435:bool)
              n282 = Less Or Equal?(x=w440, y=-500.0) -> (x <= y?=w437:bool)
              n283 = Equal To 0?(x=w442) -> (x = 0?=w438:bool)
              n284 = Compound Arithmetic op=OR(w438, w437, w435) -> (w436:bool)
            }
          }
          frame #8 {
            n285 = while {
              tunnel: w443 -> [w448]
              stop <- w444 stop-if-true
              n286 = call "PCI1220U停止.vi"("AxisHandle IN"=w448) -> ("完成"=w445:bool)  [unwired: 9 in, 1 out]
              n287 = local read "循环退出"() -> (w446:bool)
              n288 = Wait (ms)(milliseconds to wait=u32 50 ("毫秒倍数")) -> ()  [unwired: 1 out]
              n289 = Compound Arithmetic op=OR(w445, w446) -> (w444:bool)
            }
          }
          frame #9 {
            n290 = local read "电动缸快速"() -> (w449:dbl)
            n291 = local write "电动缸速度(mm/s)"(w449) -> ()
            n292 = Wait (ms)(milliseconds to wait=u32 100 ("毫秒倍数")) -> ()  [unwired: 1 out]
          }
          frame #10 {
            n293 = while {
              tunnel: w453 -> [w461]
              tunnel: [w459] -> w452
              stop <- w455 stop-if-true
              n294 = local read "齿条右极限"() -> (w458:dbl)
              n295 = Wait (ms)(milliseconds to wait=u32 50 ("毫秒倍数")) -> ()  [unwired: 1 out]
              n296 = local read "循环退出"() -> (w457:bool)
              n297 = call "PCI1240电动缸位置模式 .vi"("Distance"=w458, "AxisHandle IN"=w461) -> ("AbsSuccess"=w456:bool, "AxisHandle OUT"=w459:u32)  [unwired: 8 in]
              n298 = Compound Arithmetic op=OR(w456, w457) -> (w455:bool)
            }
            n299 = local read "转向器中心"() -> (w454:dbl)
          }
          frame #11 {
            w466 = dbl[] []
            n300 = while {
              shift-right: [w485] -> w464
              shift-left: w466 -> [w495]
              shift-right: [w493] -> w465
              shift-left: w466 -> [w494]
              tunnel: w462 -> [w489]
              tunnel: w467 -> [w488]
              shift-right: [w484] -> w463
              shift-left: w466 -> [w486]
              stop <- w478 stop-if-true
              n301 = local read "中间位置间隙"() -> (w475:dbl)
              n302 = local read "基准位移"() -> (w490:dbl)
              n303 = local read "间隙位移(mm)"() -> (w474:dbl)
              n304 = local read "电动缸位置(mm)"() -> (w470:dbl)
              n305 = call <userlib>:"Acm_AxGetCmdVelocity.vi"("AxisHandle"=w489) -> ("Velocity"=w483:dbl)  [unwired: 1 in, 3 out]
              n306 = Wait (ms)(milliseconds to wait=u32 50 ("毫秒倍数")) -> ()  [unwired: 1 out]
              n307 = disable-structure shown="禁用" {
                disable-tunnel: w474 -> [w502 _]
                frame Disabled {
                  n308 = Less Or Equal?(x=w502, y=-1.0) -> (x <= y?=w501:bool)
                  n309 = Greater Or Equal?(x=w502, y=4.0) -> (x >= y?=w500:bool)
                  n310 = Or(x=w500, y=w501) -> (x .or. y?=w499:bool)
                  n311 = property on="间隙位移(mm)" class="DigNum (严格)"("Blinking"=w499) -> ()  [unwired: 2 in, 2 out]
                }
                frame Enabled {
                }
              }
              n312 = local read "齿条推拉力(N)"() -> (w481:dbl)
              n313 = Subtract(x=w474, y=w490) -> (x-y=w477:dbl)
              n314 = Subtract(x=w477, y=w475) -> (x-y=w476:dbl)
              n315 = Subtract(x=w470, y=w488) -> (x-y=w473:dbl)
              n316 = Negate(x=w476) -> (-x=w468:dbl)
              n317 = local read "循环退出"() -> (w469:bool)
              n318 = Multiply(x=w473, y=1.0) -> (x*y=w471:dbl)
              n319 = Build Array (concatenate) ("创建数组")(w494, w468) -> (w493:dbl[])
              n320 = Build Array (concatenate) ("创建数组")(w495, w471) -> (w485:dbl[])
              n321 = Build Array (concatenate) ("创建数组")(w486, w481) -> (w484:dbl[])
              n322 = Greater Or Equal?(x=w481, y=500.0) -> (x >= y?=w479:bool)
              n323 = Equal To 0?(x=w483) -> (x = 0?=w480:bool)
              n324 = Bundle ("捆绑")(w485, w493) -> (w491:cluster{dbl[], dbl[]})  [unwired: 1 in]
              n325 = Compound Arithmetic op=OR(w480, w479, w469) -> (w478:bool)
              n326 = Bundle ("捆绑")(w485, w484) -> (w487:cluster{dbl[], dbl[]})  [unwired: 1 in]
              n327 = Build Array ("创建数组")(w491, w487) -> (w492:cluster{dbl[], dbl[]}[])
              n328 = local write "行程跳动曲线"(w492) -> ()
            }
          }
          frame #12 {
            n329 = local read "电动缸慢速"() -> (w503:dbl)
            n330 = local write "电动缸速度(mm/s)"(w503) -> ()
          }
          frame #13 {
            n331 = while {
              tunnel: w513 -> [w520]
              tunnel: [w518] -> w509
              stop <- w515 stop-if-true
              n332 = Wait (ms)(milliseconds to wait=u32 50 ("毫秒倍数")) -> ()  [unwired: 1 out]
              n333 = local read "循环退出"() -> (w517:bool)
              n334 = call "PCI1240电动缸位置模式 .vi"("Distance"=-20.0, "AxisHandle IN"=w520) -> ("AbsSuccess"=w516:bool, "AxisHandle OUT"=w518:u32)  [unwired: 8 in]
              n335 = Compound Arithmetic op=OR(w516, w517) -> (w515:bool)
            }
            n336 = local read "转向器中心"() -> (w508:dbl)
          }
          frame #14 {
            n337 = while {
              shift-right: [w546] -> w527
              shift-left: w524 -> [w556]
              shift-right: [w554] -> w528
              shift-left: w525 -> [w555]
              tunnel: w521 -> [w550]
              tunnel: w522 -> [w549]
              shift-right: [w545] -> w526
              shift-left: w523 -> [w547]
              stop <- w539 stop-if-true
              n338 = local read "中间位置间隙"() -> (w536:dbl)
              n339 = local read "基准位移"() -> (w551:dbl)
              n340 = local read "间隙位移(mm)"() -> (w535:dbl)
              n341 = local read "电动缸位置(mm)"() -> (w531:dbl)
              n342 = call <userlib>:"Acm_AxGetCmdVelocity.vi"("AxisHandle"=w550) -> ("Velocity"=w544:dbl)  [unwired: 1 in, 3 out]
              n343 = Wait (ms)(milliseconds to wait=u32 50 ("毫秒倍数")) -> ()  [unwired: 1 out]
              n344 = disable-structure shown="禁用" {
                disable-tunnel: w535 -> [w563 _]
                frame Disabled {
                  n345 = Less Or Equal?(x=w563, y=-1.0) -> (x <= y?=w562:bool)
                  n346 = Greater Or Equal?(x=w563, y=4.0) -> (x >= y?=w561:bool)
                  n347 = Or(x=w561, y=w562) -> (x .or. y?=w560:bool)
                  n348 = property on="间隙位移(mm)" class="DigNum (严格)"("Blinking"=w560) -> ()  [unwired: 2 in, 2 out]
                }
                frame Enabled {
                }
              }
              n349 = local read "齿条推拉力(N)"() -> (w542:dbl)
              n350 = Subtract(x=w535, y=w551) -> (x-y=w538:dbl)
              n351 = Subtract(x=w531, y=w549) -> (x-y=w534:dbl)
              n352 = Subtract(x=w538, y=w536) -> (x-y=w537:dbl)
              n353 = Negate(x=w537) -> (-x=w529:dbl)
              n354 = Multiply(x=w534, y=1.0) -> (x*y=w532:dbl)
              n355 = local read "循环退出"() -> (w530:bool)
              n356 = Build Array (concatenate) ("创建数组")(w555, w529) -> (w554:dbl[])
              n357 = Build Array (concatenate) ("创建数组")(w556, w532) -> (w546:dbl[])
              n358 = Build Array (concatenate) ("创建数组")(w547, w542) -> (w545:dbl[])
              n359 = Greater Or Equal?(x=w542, y=500.0) -> (x >= y?=w540:bool)
              n360 = Equal To 0?(x=w544) -> (x = 0?=w541:bool)
              n361 = Bundle ("捆绑")(w546, w554) -> (w552:cluster{dbl[], dbl[]})  [unwired: 1 in]
              n362 = Bundle ("捆绑")(w546, w545) -> (w548:cluster{dbl[], dbl[]})  [unwired: 1 in]
              n363 = Compound Arithmetic op=OR(w541, w540, w530) -> (w539:bool)
              n364 = Build Array ("创建数组")(w552, w548) -> (w553:cluster{dbl[], dbl[]}[])
              n365 = local write "行程跳动曲线"(w553) -> ()
            }
          }
          frame #15 {
            n366 = while {
              tunnel: w580 -> [w587]
              tunnel: [w586] -> _
              stop <- w582 stop-if-true
              n367 = call "PCI1220U停止.vi"("AxisHandle IN"=w587) -> ("完成"=w583:bool, "AxisHandle OUT"=w586:u32)  [unwired: 9 in]
              n368 = Wait (ms)(milliseconds to wait=u32 50 ("毫秒倍数")) -> ()  [unwired: 1 out]
              n369 = local read "循环退出"() -> (w584:bool)
              n370 = Compound Arithmetic op=OR(w583, w584) -> (w582:bool)
            }
            n371 = call "功能计算_何 截取位移左.vi"("位移数组"=w566, "拉压力数组"=w579, "半行程"="半行程", "截取百分比"="截取百分比") -> ("峰值扭矩"=w578:dbl, "平均扭矩"=w577:dbl, "扭差"=w576:dbl)  [unwired: 12 in, 1 out]
            "左轴向力波动(N)" <- w576
            "左最大轴向力(N)" <- w578
            n372 = call "间隙计算.vi"("扭矩数组"=w581) -> ("峰值间隙1"=w575:dbl, "峰值间隙2"=w574:dbl)  [unwired: 6 in, 3 out]
            n373 = local read "180°内全行程间隙标准(mm)"() -> (w573:dbl)
            n374 = Array Size(array=w566) -> (size(s)=w565:i32)
            n375 = local read "180°外全行程间隙标准(mm)"() -> (w570:dbl)
            n376 = local write "左平均轴向力(N)"(w577) -> ()
            n377 = local write "左180°外全行程间隙"(w574) -> ()
            n378 = local write "左180°内全行程间隙"(w575) -> ()
            n379 = local write "左轴向力数组大小"(w565) -> ()
            n380 = local read "电动缸快速"() -> (w564:dbl)
            n381 = Greater?(x=w575, y=w573) -> (0:w572:bool)
            n382 = Greater?(x=w574, y=w570) -> (0:w571:bool)
            n383 = property on="左180°内全行程间隙" class="DigNum (严格)"("Blinking"=w572) -> ()  [unwired: 2 in, 2 out]
            n384 = property on="左180°外全行程间隙" class="DigNum (严格)"("Blinking"=w571) -> ()  [unwired: 2 in, 2 out]
            n385 = local write "电动缸速度(mm/s)"(w564) -> ()
            n386 = local read "最大轴向力标准(N)"() -> (w567:dbl)
          }
          frame #16 {
            n387 = while {
              tunnel: w601 -> [w610]
              tunnel: [w608] -> w590
              stop <- w605 stop-if-true
              n388 = Wait (ms)(milliseconds to wait=u32 50 ("毫秒倍数")) -> ()  [unwired: 1 out]
              n389 = local read "循环退出"() -> (w607:bool)
              n390 = call "PCI1240电动缸位置模式 .vi"("Distance"=150.0, "AxisHandle IN"=w610) -> ("AbsSuccess"=w606:bool, "AxisHandle OUT"=w608:u32)  [unwired: 8 in]
              n391 = Compound Arithmetic op=OR(w606, w607) -> (w605:bool)
            }
            n392 = local read "轴向力标准(N)"() -> (w595:dbl)
            n393 = local read "平均轴向力标准(N) max"() -> (w594:dbl)
            n394 = local read "力波动标准(N)"() -> (w593:dbl)
            n395 = call "判断.vi"("y 3"=w593, "y 2-2"=w594, "y 2-1"=w595, "y"=w588, "x 3"=w598, "x 2"=w599, "x"=w597) -> ("非x? 3"=w591:bool, "非x? 2"=w596:bool, "非x?"=w592:bool)  [unwired: 2 in]
            n396 = property on="左最大轴向力(N)" class="DigNum (严格)"("Blinking"=w592) -> ()  [unwired: 2 in, 2 out]
            n397 = property on="左平均轴向力(N)" class="DigNum (严格)"("Blinking"=w596) -> ()  [unwired: 2 in, 2 out]
            n398 = property on="左轴向力波动(N)" class="DigNum (严格)"("Blinking"=w591) -> ()  [unwired: 2 in, 2 out]
            n399 = local read "转向器中心"() -> (w589:dbl)
          }
          frame #17 {
            n400 = while {
              shift-right: [w646] -> w612
              shift-left: w615 -> [w655]
              shift-right: [w653] -> w614
              shift-left: w616 -> [w654]
              tunnel: w611 -> [w648]
              tunnel: w618 -> [w647]
              shift-right: [w643] -> w613
              shift-left: w617 -> [w644]
              stop <- w638 stop-if-true
              n401 = local read "电动缸位置(mm)"() -> (w623:dbl)
              n402 = call <userlib>:"Acm_AxGetCmdVelocity.vi"("AxisHandle"=w648) -> ("Velocity"=w636:dbl)  [unwired: 1 in, 3 out]
              n403 = local read "间隙位移(mm)"() -> (w630:dbl)
              n404 = local read "基准位移"() -> (w649:dbl)
              n405 = Wait (ms)(milliseconds to wait=u32 50 ("毫秒倍数")) -> ()  [unwired: 1 out]
              n406 = local read "中间位置间隙"() -> (w635:dbl)
              n407 = local read "齿条推拉力(N)"() -> (w642:dbl)
              n408 = Add(x=1.47, y=w623) -> (x+y=w625:dbl)
              n409 = Subtract(x=w630, y=w649) -> (x-y=w650:dbl)
              n410 = Subtract(x=w625, y=w647) -> (x-y=w628:dbl)
              n411 = local read "循环退出"() -> (w622:bool)
              n412 = Subtract(x=w650, y=w635) -> (x-y=w637:dbl)
              n413 = Negate(x=w637) -> (-x=w621:dbl)
              n414 = Multiply(x=w628, y=1.0) -> (x*y=w626:dbl)
              n415 = Build Array (concatenate) ("创建数组")(w655, w626) -> (w646:dbl[])
              n416 = Less Or Equal?(x=w642, y=-500.0) -> (x <= y?=w639:bool)
              n417 = Build Array (concatenate) ("创建数组")(w644, w642) -> (w643:dbl[])
              n418 = Equal To 0?(x=w636) -> (x = 0?=w640:bool)
              n419 = Build Array (concatenate) ("创建数组")(w654, w621) -> (w653:dbl[])
              n420 = Bundle ("捆绑")(w646, w643) -> (w645:cluster{dbl[], dbl[]})  [unwired: 1 in]
              n421 = Compound Arithmetic op=OR(w640, w639, w622) -> (w638:bool)
              n422 = Bundle ("捆绑")(w646, w653) -> (w651:cluster{dbl[], dbl[]})  [unwired: 1 in]
              n423 = Build Array ("创建数组")(w651, w645) -> (w652:cluster{dbl[], dbl[]}[])
              n424 = Less Or Equal?(x=w630, y=-1.0) -> (x <= y?=w634:bool)
              n425 = Greater Or Equal?(x=w630, y=4.0) -> (x >= y?=w633:bool)
              n426 = local write "行程跳动曲线"(w652) -> ()
              n427 = Or(x=w633, y=w634) -> (x .or. y?=w629:bool)
              n428 = disable-structure shown="禁用" {
                disable-tunnel: w629 -> [w657 _]
                frame Disabled {
                  n429 = property on="间隙位移(mm)" class="DigNum (严格)"("Blinking"=w657) -> ()  [unwired: 2 in, 2 out]
                }
                frame Enabled {
                }
              }
            }
          }
          frame #18 {
            n430 = local read "电动缸慢速"() -> (w658:dbl)
            n431 = local write "电动缸速度(mm/s)"(w658) -> ()
          }
          frame #19 {
            n432 = while {
              tunnel: w666 -> [w678]
              stop <- w673 stop-if-true
              n433 = Wait (ms)(milliseconds to wait=u32 50 ("毫秒倍数")) -> ()  [unwired: 1 out]
              n434 = local read "循环退出"() -> (w675:bool)
              n435 = call "PCI1240电动缸位置模式 .vi"("Distance"=160.0, "AxisHandle IN"=w678) -> ("AbsSuccess"=w674:bool)  [unwired: 8 in, 1 out]
              n436 = Compound Arithmetic op=OR(w674, w675) -> (w673:bool)
            }
          }
          frame #20 {
            n437 = while {
              shift-right: [w714] -> w687
              shift-left: w681 -> [w723]
              shift-right: [w721] -> w688
              shift-left: w680 -> [w722]
              tunnel: w679 -> [w716]
              tunnel: w682 -> [w715]
              shift-right: [w711] -> w686
              shift-left: w683 -> [w712]
              stop <- w706 stop-if-true
              n438 = local read "电动缸位置(mm)"() -> (w691:dbl)
              n439 = call <userlib>:"Acm_AxGetCmdVelocity.vi"("AxisHandle"=w716) -> ("Velocity"=w704:dbl)  [unwired: 1 in, 3 out]
              n440 = local read "间隙位移(mm)"() -> (w698:dbl)
              n441 = local read "基准位移"() -> (w717:dbl)
              n442 = Wait (ms)(milliseconds to wait=u32 50 ("毫秒倍数")) -> ()  [unwired: 1 out]
              n443 = local read "中间位置间隙"() -> (w703:dbl)
              n444 = local read "齿条推拉力(N)"() -> (w710:dbl)
              n445 = Subtract(x=w698, y=w717) -> (x-y=w718:dbl)
              n446 = Add(x=1.45, y=w691) -> (x+y=w693:dbl)
              n447 = Subtract(x=w693, y=w715) -> (x-y=w696:dbl)
              n448 = Subtract(x=w718, y=w703) -> (x-y=w705:dbl)
              n449 = local read "循环退出"() -> (w690:bool)
              n450 = Negate(x=w705) -> (-x=w689:dbl)
              n451 = Multiply(x=w696, y=1.0) -> (x*y=w694:dbl)
              n452 = Build Array (concatenate) ("创建数组")(w723, w694) -> (w714:dbl[])
              n453 = Less Or Equal?(x=w710, y=-500.0) -> (x <= y?=w707:bool)
              n454 = Build Array (concatenate) ("创建数组")(w712, w710) -> (w711:dbl[])
              n455 = Equal To 0?(x=w704) -> (x = 0?=w708:bool)
              n456 = Build Array (concatenate) ("创建数组")(w722, w689) -> (w721:dbl[])
              n457 = Bundle ("捆绑")(w714, w711) -> (w713:cluster{dbl[], dbl[]})  [unwired: 1 in]
              n458 = Compound Arithmetic op=OR(w708, w707, w690) -> (w706:bool)
              n459 = Bundle ("捆绑")(w714, w721) -> (w719:cluster{dbl[], dbl[]})  [unwired: 1 in]
              n460 = Build Array ("创建数组")(w719, w713) -> (w720:cluster{dbl[], dbl[]}[])
              n461 = Less Or Equal?(x=w698, y=-1.0) -> (x <= y?=w702:bool)
              n462 = Greater Or Equal?(x=w698, y=4.0) -> (x >= y?=w701:bool)
              n463 = local write "行程跳动曲线"(w720) -> ()
              n464 = Or(x=w701, y=w702) -> (x .or. y?=w697:bool)
              n465 = disable-structure shown="禁用" {
                disable-tunnel: w697 -> [w725 _]
                frame Disabled {
                  n466 = property on="间隙位移(mm)" class="DigNum (严格)"("Blinking"=w725) -> ()  [unwired: 2 in, 2 out]
                }
                frame Enabled {
                }
              }
            }
          }
          frame #21 {
            n467 = while {
              tunnel: w734 -> [w743]
              tunnel: [w742] -> _
              stop <- w738 stop-if-true
              n468 = local read "循环退出"() -> (w740:bool)
              n469 = call "PCI1220U停止.vi"("AxisHandle IN"=w743) -> ("完成"=w739:bool, "AxisHandle OUT"=w742:u32)  [unwired: 9 in]
              n470 = Wait (ms)(milliseconds to wait=u32 50 ("毫秒倍数")) -> ()  [unwired: 1 out]
              n471 = Compound Arithmetic op=OR(w739, w740) -> (w738:bool)
            }
            n472 = Array Max & Min(array=w731) -> (max value=w733:dbl, min value=w732:dbl)  [unwired: 2 out]
            n473 = local read "左轴向力数组大小"() -> (w726:i32)
            n474 = Absolute Value(x=w733) -> (abs(x)=w730:dbl)
            n475 = Absolute Value(x=w732) -> (abs(x)=w729:dbl)
            n476 = local write "左全行程间隙"(w730) -> ()
            n477 = local write "右全行程间隙"(w729) -> ()
          }
          frame #22 {
            n478 = local read "180°内全行程间隙标准(mm)"() -> (w775:dbl)
            n479 = local read "截取百分比"() -> (w748:dbl)
            n480 = local read "齿条传动比"() -> (w752:dbl)
            n481 = local read "半行程"() -> (w749:dbl)
            n482 = Split 1D Array(array=w782, index=w744) -> (second subarray=w781:dbl[])  [unwired: 1 out]
            n483 = Split 1D Array(array=w750, index=w744) -> (second subarray=w751:dbl[])  [unwired: 1 out]
            n484 = Array Max & Min(array=w750) -> (max value=w771:dbl, min value=w770:dbl)  [unwired: 2 out]
            n485 = local read "机械间隙值"() -> (w764:dbl)
            n486 = local read "总圈数标准"() -> (w756:dbl)
            n487 = local read "总圈数最大值"() -> (w757:dbl)
            n488 = Subtract(x=w771, y=w770) -> (x-y=w765:dbl)
            n489 = call "功能计算_何 截取位移右.vi"("位移数组"=w751, "拉压力数组"=w781, "半行程"=w749, "截取百分比"=w748) -> ("峰值扭矩"=w747:dbl, "平均扭矩"=w780:dbl, "扭差"=w746:dbl)  [unwired: 12 in, 1 out]
            "右最大轴向力(N)" <- w747
            "右轴向力波动(N)" <- w746
            n490 = Subtract(x=w765, y=w764) -> (x-y=w762:dbl)
            n491 = Split 1D Array(array=w779, index=w744) -> (second subarray=w778:dbl[])  [unwired: 1 out]
            n492 = Greater?(x=w777, y=w775) -> (0:w767:bool)
            n493 = Greater?(x=w776, y=w775) -> (0:w766:bool)
            n494 = call "间隙计算.vi"("扭矩数组"=w778) -> ("峰值间隙1"=w773:dbl, "峰值间隙2"=w772:dbl)  [unwired: 6 in, 3 out]
            n495 = Divide(x=w762, y=w752) -> (x/y=w755:dbl)
            n496 = In Range and Coerce(upper limit=w757, x=w755, lower limit=w756) -> (In Range?=w754:bool)  [unwired: 1 out]
            n497 = Not(x=w754) -> (.not. x?=w753:bool)
            n498 = property on="总圈数" class="DigNum (严格)"("Blinking"=w753) -> ()  [unwired: 2 in, 2 out]
            n499 = property on="左全行程间隙" class="DigNum (严格)"("Blinking"=w767) -> ()  [unwired: 2 in, 2 out]
            n500 = property on="右全行程间隙" class="DigNum (严格)"("Blinking"=w766) -> ()  [unwired: 2 in, 2 out]
            n501 = local write "右平均轴向力(N)"(w780) -> ()
            n502 = local write "总圈数"(w755) -> ()
            n503 = local read "180°内全行程间隙标准(mm)"() -> (w774:dbl)
            n504 = local read "总行程标准(mm)"() -> (w760:dbl)
            n505 = local read "总行程最大值"() -> (w761:dbl)
            n506 = In Range and Coerce(upper limit=w761, x=w762, lower limit=w760) -> (In Range?=w759:bool)  [unwired: 1 out]
            n507 = local write "右180°外全行程间隙"(w772) -> ()
            n508 = local write "右180°内全行程间隙"(w773) -> ()
            n509 = local read "180°外全行程间隙标准(mm)"() -> (w763:dbl)
            n510 = local read "最大轴向力标准(N)"() -> (w745:dbl)
            n511 = Not(x=w759) -> (.not. x?=w758:bool)
            n512 = local write "总行程"(w762) -> ()
            n513 = property on="总行程" class="DigNum (严格)"("Blinking"=w758) -> ()  [unwired: 2 in, 2 out]
            "轴向力X" <- w750
            "轴向力Y" <- w782
          }
          frame #23 {
            n514 = local read "电动缸快速"() -> (w785:dbl)
            n515 = local read "轴向力标准(N)"() -> (w799:dbl)
            n516 = local read "平均轴向力标准(N) max"() -> (w798:dbl)
            n517 = Greater?(x=w805, y=w806) -> (0:w791:bool)
            n518 = Greater?(x=w804, y=w789) -> (0:w790:bool)
            n519 = local write "电动缸速度(mm/s)"(w785) -> ()
            n520 = local read "转向器中心"() -> (w807:dbl)
            n521 = local read "力波动标准(N)"() -> (w797:dbl)
            n522 = call "判断.vi"("y 3"=w797, "y 2-2"=w798, "y 2-1"=w799, "y"=w786, "x 3"=w800, "x 2"=w810, "x"=w801) -> ("非x? 3"=w794:bool, "非x? 2"=w802:bool, "非x?"=w803:bool)  [unwired: 2 in]
            n523 = property on="右180°内全行程间隙" class="DigNum (严格)"("Blinking"=w791) -> ()  [unwired: 2 in, 2 out]
            n524 = property on="右180°外全行程间隙" class="DigNum (严格)"("Blinking"=w790) -> ()  [unwired: 2 in, 2 out]
            n525 = Add(x=w807, y=0.0) -> (x+y=w808:dbl)
          }
          frame #24 {
            n526 = Compound Arithmetic op=OR(w819, w818, w817, w816) -> (w815:bool)
            n527 = property on="右最大轴向力(N)" class="DigNum (严格)"("Blinking"=w822) -> ()  [unwired: 2 in, 2 out]
            n528 = property on="右平均轴向力(N)" class="DigNum (严格)"("Blinking"=w821) -> ()  [unwired: 2 in, 2 out]
            n529 = property on="右轴向力波动(N)" class="DigNum (严格)"("Blinking"=w820) -> ()  [unwired: 2 in, 2 out]
            n530 = Compound Arithmetic op=OR(w813, w815, w822, w820, w824, w823, w814) -> (w826:bool)
            n531 = Not(x=w826) -> (.not. x?=w825:bool)
            n532 = local write "轴向力及全行程间隙合格"(w825) -> ()
            n533 = Wait (ms)(milliseconds to wait=u32 100 ("等待时间（毫秒）")) -> ()  [unwired: 1 out]
          }
          frame #25 {
            n534 = while {
              tunnel: w831 -> [w835]
              tunnel: [w833] -> w830
              tunnel: w829 -> [w832]
              stop <- w834 stop-if-true
              n535 = call "PCI1240电动缸位置模式 .vi"("Distance"=w832, "AxisHandle IN"=w835) -> ("AbsSuccess"=w834:bool, "AxisHandle OUT"=w833:u32)  [unwired: 8 in]
              n536 = Wait (ms)(milliseconds to wait=u32 50 ("毫秒倍数")) -> ()  [unwired: 1 out]
            }
          }
          frame #26 {
            n537 = while {
              tunnel: w838 -> [w843]
              tunnel: [w839] -> w837
              stop <- w841 stop-if-true
              n538 = call <userlib>:"Acm_AxGetCmdVelocity.vi"("AxisHandle"=w843) -> ("Velocity"=w842:dbl, "AxisHandle"=w839:u32)  [unwired: 1 in, 2 out]
              n539 = Wait Until Next ms Multiple(millisecond multiple=u32 50 ("毫秒倍数")) -> ()  [unwired: 1 out]
              n540 = Equal To 0?(x=w842) -> (x = 0?=w841:bool)
            }
          }
          frame #27 {
            n541 = call "PCI1220U停止.vi"("AxisHandle IN"=w844) -> ()  [unwired: 9 in, 2 out]
          }
          frame #28 {
          }
          frame #29 {
            n542 = local read "轴向力已做次数"() -> (w847:dbl)
            n543 = Add(x=w847, y=1.0) -> (x+y=w845:dbl)
            n544 = local write "轴向力已做次数"(w845) -> ()
          }
          frame #30 {
            n545 = local read "轴向力及全行程间隙合格"() -> (w848:bool)
            n546 = case shown="假" w848 {
              frame False {
                n547 = Less?(x="轴向力已做次数", y="轴向力设定次数") -> (x < y?=w850:bool)
                n548 = case shown="真" w850 {
                  frame False {
                    n549 = local write "工步号"(u32 45 ("工步号")) -> ()
                  }
                  frame True {
                    n550 = local write "工步号"(u32 30 ("工步号")) -> ()
                  }
                }
              }
              frame True {
                n551 = local write "工步号"(u32 45 ("工步号")) -> ()
              }
            }
          }
        }
      }
      frame 45 {
        # "测头退回"
        n552 = flat-sequence {
          tunnel: [w858] -> w855
          tunnel: w855 -> [w865]
          frame #0 {
            n553 = local write "测头机构轴速度(mm/s)"(30.0 ("测头机构轴速度(mm/s)")) -> ()
          }
          frame #1 {
            n554 = local read "测头机构轴后退位"() -> (w857:dbl)
            n555 = local read "测头机构电机"() -> (w859:u32)
            n556 = while {
              tunnel: w859 -> [w863]
              tunnel: w857 -> [w862]
              tunnel: [w861] -> w858
              stop <- w864 stop-if-true
              n557 = Wait Until Next ms Multiple(millisecond multiple=u32 50 ("毫秒倍数")) -> ()  [unwired: 1 out]
              n558 = call "PCI1220U进给轴位置模式.vi"("Distance"=w862, "AxisHandle IN"=w863) -> ("AbsSuccess"=w864:bool, "AxisHandle OUT"=w861:u32)  [unwired: 8 in]
            }
          }
          frame #2 {
            n559 = while {
              tunnel: w865 -> [w869]
              stop <- w867 stop-if-true
              n560 = call <userlib>:"Acm_AxGetCmdVelocity.vi"("AxisHandle"=w869) -> ("Velocity"=w868:dbl)  [unwired: 1 in, 3 out]
              n561 = Wait Until Next ms Multiple(millisecond multiple=u32 50 ("毫秒倍数")) -> ()  [unwired: 1 out]
              n562 = Equal To 0?(x=w868) -> (x = 0?=w867:bool)
            }
          }
          frame #3 {
            n563 = while {
              stop <- w871 stop-if-true
              n564 = local read "测头机构轴位置(mm)"() -> (w873:dbl)
              n565 = Wait Until Next ms Multiple(millisecond multiple=u32 50 ("毫秒倍数")) -> ()  [unwired: 1 out]
              n566 = Less Or Equal?(x=w873, y=35.0) -> (x <= y?=w871:bool)
            }
          }
          frame #4 {
            n567 = local write "测头气缸右移"(FALSE ("测头气缸右移")) -> ()
            n568 = local write "测头气缸左移"(TRUE ("测头气缸左移")) -> ()
          }
          frame #5 {
            n569 = Wait Until Next ms Multiple(millisecond multiple=u32 500 ("毫秒倍数")) -> ()  [unwired: 1 out]
          }
          frame #6 {
            n570 = local write "工步号"(u32 50 ("工步号")) -> ()
          }
        }
      }
      frame 50 {
        n571 = flat-sequence {
          tunnel: [w890] -> w879
          tunnel: w879 -> [w897]
          tunnel: [w896] -> w878
          tunnel: w878 -> [w908]
          frame #0 {
            n572 = local write "夹头夹紧"(FALSE ("夹头夹紧")) -> ()
            n573 = local write "夹头松开"(TRUE ("夹头松开")) -> ()
            n574 = local write "测头机构轴速度(mm/s)"(15.0 ("调整机构轴速度(mm/s)")) -> ()
            n575 = local write "电动缸速度(mm/s)"(15.0 ("电动缸速度(mm/s)")) -> ()
          }
          frame #1 {
            n576 = while {
              stop <- w884 stop-if-true
              n577 = local read "夹头夹紧"() -> (w887:bool)
              n578 = Wait Until Next ms Multiple(millisecond multiple=u32 50 ("毫秒倍数")) -> ()  [unwired: 1 out]
              n579 = local read "夹头松开"() -> (w885:bool)
              n580 = Not(x=w887) -> (.not. x?=w886:bool)
              n581 = And(x=w886, y=w885) -> (x .and. y?=w884:bool)
            }
          }
          frame #2 {
            n582 = Wait (ms)(milliseconds to wait=u32 1000 ("等待时间（毫秒）")) -> ()  [unwired: 1 out]
          }
          frame #3 {
            n583 = while {
              tunnel: [w893] -> w890
              stop <- w892 stop-if-true
              n584 = local read "电动缸电机"() -> (w894:u32)
              n585 = Wait Until Next ms Multiple(millisecond multiple=u32 50 ("毫秒倍数")) -> ()  [unwired: 1 out]
              n586 = call "PCI1240电动缸位置模式 .vi"("Distance"=0.0, "AxisHandle IN"=w894) -> ("AbsSuccess"=w892:bool, "AxisHandle OUT"=w893:u32)  [unwired: 8 in]
            }
          }
          frame #4 {
            n587 = while {
              tunnel: w897 -> [w906]
              tunnel: [w898] -> w896
              stop <- w899 stop-if-true
              n588 = local read "齿条推拉力(N)"() -> (w904:dbl)
              n589 = Wait Until Next ms Multiple(millisecond multiple=u32 50 ("毫秒倍数")) -> ()  [unwired: 1 out]
              n590 = Absolute Value(x=w904) -> (abs(x)=w903:dbl)
              n591 = call <userlib>:"Acm_AxGetCmdVelocity.vi"("AxisHandle"=w906) -> ("Velocity"=w907:dbl, "AxisHandle"=w898:u32)  [unwired: 1 in, 2 out]
              n592 = Greater Or Equal?(x=w903, y=1000.0) -> (x >= y?=w900:bool)
              n593 = Equal To 0?(x=w907) -> (x = 0?=w901:bool)
              n594 = Or(x=w901, y=w900) -> (x .or. y?=w899:bool)
            }
          }
          frame #5 {
            n595 = while {
              tunnel: w908 -> [w911]
              stop <- w910 stop-if-true
              n596 = call "PCI1220U停止.vi"("AxisHandle IN"=w911) -> ("完成"=w910:bool)  [unwired: 9 in, 1 out]
              n597 = Wait (ms)(milliseconds to wait=u32 50 ("毫秒倍数")) -> ()  [unwired: 1 out]
            }
          }
          frame #6 {
            n598 = local write "工步号"(u32 100 ("工步号")) -> ()
          }
        }
      }
      frame 100 {
        n599 = flat-sequence {
          tunnel: [w946] -> w936
          tunnel: [w944] -> w935
          tunnel: [w938] -> w923
          tunnel: [w937] -> w920
          tunnel: w936 -> [w953]
          tunnel: w935 -> [w950]
          tunnel: ["F:\\报表存储\\" ("字符串")] -> w934
          tunnel: w923 -> [w952]
          tunnel: [w953] -> w922
          tunnel: [w952] -> w921
          tunnel: w920 -> [w951]
          tunnel: [w951] -> w919
          tunnel: [w950] -> w918
          tunnel: w934 -> [w965]
          tunnel: [w972] -> w933
          tunnel: [w970] -> w932
          tunnel: [w969] -> w931
          tunnel: [w968] -> w930
          tunnel: w922 -> [w964]
          tunnel: w921 -> [w963]
          tunnel: w919 -> [w962]
          tunnel: w918 -> [w955]
          tunnel: [w957] -> w913
          tunnel: w933 -> [w979]
          tunnel: [w980] -> w929
          tunnel: w932 -> [w980]
          tunnel: w931 -> [w978]
          tunnel: w930 -> [w977]
          tunnel: [w976] -> w928
          tunnel: [w975] -> w927
          tunnel: [w974] -> w914
          tunnel: w913 -> [w974]
          tunnel: [w987] -> w926
          tunnel: w929 -> [w987]
          tunnel: w928 -> [w986]
          tunnel: [w986] -> w925
          tunnel: [w985] -> w924
          tunnel: w927 -> [w985]
          tunnel: [w983] -> w915
          tunnel: w914 -> [w983]
          tunnel: w926 -> [w990]
          tunnel: w925 -> [w998]
          tunnel: w924 -> [w997]
          tunnel: [w989] -> w916
          tunnel: w915 -> [w989]
          tunnel: [w1006] -> w917
          tunnel: w916 -> [w1006]
          tunnel: w917 -> [w1008]
          frame #0 {
            n600 = local read "产品ID"() -> (w945:string)
            n601 = Format Date/Time String(time format string (%c)="%Y%m%d" ("时间格式字符串(%c)")) -> (date/time string=w939:string)  [unwired: 2 in]
            n602 = String Subset(string=w939, offset (0)=6 ("偏移量(0)"), length (rest)=2 ("长度（剩余）")) -> (substring=w937:string)
            n603 = String Subset(string=w939, offset (0)=4 ("偏移量(0)"), length (rest)=2 ("长度（剩余）")) -> (substring=w938:string)
            n604 = String Subset(string=w939, offset (0)=0 ("偏移量(0)"), length (rest)=4 ("长度（剩余）")) -> (substring=w946:string)
            n605 = call <vilib>:"Trim Whitespace.vi"("string"=w945) -> ("trimmed string"=w944:string)  [unwired: 1 in]
          }
          frame #1 {
          }
          frame #2 {
            w956 = "\\" ("字符串")
            n606 = Concatenate Strings(w965, w964, w956, w963, w956, w962, w956, w955, w956) -> (w959:string)
            n607 = Concatenate Strings(w965, w964, w956, w963, w956, w962, w956, w955, w956) -> (w973:string)
            n608 = Concatenate Strings(w959, w955, "间隙曲线.JPG" ("字符串")) -> (w971:string)
            n609 = Concatenate Strings(w959, "轴向力曲线数组.txt" ("字符串")) -> (w968:string)
            n610 = Concatenate Strings(w959, "扭动曲线数组.txt" ("字符串")) -> (w969:string)
            n611 = Concatenate Strings(w959, w955, "轴向力曲线.JPG" ("字符串")) -> (w961:string)
            n612 = String To Path(string=w971) -> (path=w970:path)
            n613 = String To Path(string=w973) -> (path=w972:path)
            n614 = String To Path(string=w961) -> (path=w957:path)
          }
          frame #3 {
            n615 = call <vilib>:"Check if File or Folder Exists.vi"("path"=w979) -> ("file or folder exists?"=w981:bool)  [unwired: 8 in, 2 out]
            n616 = case shown="假" w981 {
              tunnel: w979 -> [w982 _]
              frame False {
                n617 = Create Folder(path (use dialog)=w982) -> ()  [unwired: 2 in, 3 out]
              }
              frame True {
              }
            }
            n618 = String To Path(string=w977) -> (path=w975:path)
            n619 = String To Path(string=w978) -> (path=w976:path)
          }
          frame #4 {
            n620 = local write "选项卡控件"(T1."间隙测量" ("选项卡控件")) -> ()
            n621 = Wait Until Next ms Multiple(millisecond multiple=u32 1000 ("毫秒倍数")) -> ()  [unwired: 1 out]
          }
          frame #5 {
            n622 = disable-structure shown="禁用" {
              disable-tunnel: w990 -> [w999 _]
              frame Disabled {
                w1003 = T2 2 items=["快速打印", "标准报表", "HTML", "双字节", "Excel"] ("report type (Quick Print)")
                w1002 = T3 1 items=["完整前面板", "前面板可见部分", "图标、说明、前面板和程序框图", "说明信息: 使用前面板", "说明信息: 作为子VI使用", "说明信息: 完整", "说明信息: 自定义"] ("contents (complete front panel)")
                n623 = Current VI's Path() -> (path=w1001:path)
                n624 = call-poly <vilib>:"Easy Print VI Panel or Documentation.vi"("report type (Quick Print)"=w1003, "contents (complete front panel)"=w1002, "VI path"=w1001) -> ("error out"=w1005:errorcluster, "report out"=w1004:refnum<class "NI_report.lvclass">)  [unwired: 1 in, 6 out]
                n625 = call-dynamic "Save Report to File.vi"("report in"=w1004, "report file path"=w999, "error in (no error)"=w1005) -> ("error out"=→"error out 3":errorcluster)  [unwired: 2 in, 10 out]
              }
              frame Enabled {
              }
            }
            n626 = local read "间隙Y数组"() -> (w995:dbl[])
            n627 = local read "间隙X数组"() -> (w996:dbl[])
            n628 = local read "轴向力Y"() -> (w993:dbl[])
            n629 = local read "轴向力X"() -> (w994:dbl[])
            n630 = call "导出曲线数组.vi"("file path (dialog if empty)"=w998, "数组 2"=w995, "数组"=w996) -> ()  [unwired: 9 in]
            n631 = call "导出曲线数组.vi"("file path (dialog if empty)"=w997, "数组 2"=w993, "数组"=w994) -> ()  [unwired: 9 in]
            n632 = control-ref of="本VI"() -> (w992:refnum<vi>)
            n633 = invoke class="VI" method="FP.Get Image"(reference=w992) -> ("image data"=w991:T4)  [unwired: 5 in, 5 out]
            n634 = call <vilib>:"Write JPEG File.vi"("image data"=w991, "path to JPEG file"=w990) -> ()  [unwired: 8 in, 2 out]
          }
          frame #6 {
            n635 = local write "选项卡控件"(T1."轴向力测量" ("选项卡控件")) -> ()
          }
          frame #7 {
            n636 = control-ref of="本VI"() -> (w1009:refnum<vi>)
            n637 = invoke class="VI" method="FP.Get Image"(reference=w1009) -> ("image data"=w1010:T4)  [unwired: 5 in, 5 out]
            n638 = call <vilib>:"Write JPEG File.vi"("image data"=w1010, "path to JPEG file"=w1008) -> ()  [unwired: 8 in, 2 out]
          }
          frame #8 {
            n639 = local read "联线按钮"() -> (w1011:bool)
            n640 = case shown="真" w1011 {
              frame False {
              }
              frame True {
                n641 = flat-sequence {
                  tunnel: [w1014] -> w1012
                  tunnel: [w1042] -> w1013
                  tunnel: w1012 -> [w1038]
                  tunnel: w1013 -> [w1054]
                  frame #0 {
                    n642 = local read "轴向力及全行程间隙合格"() -> (w1015:bool)
                    n643 = local read "单点间隙合格"() -> (w1016:bool)
                    n644 = And(x=w1016, y=w1015) -> (x .and. y?=w1014:bool)
                  }
                  frame #1 {
                    w1036 = i16 3 ("精度(6)")
                    n645 = local read "右180°内全行程间隙"() -> (w1035:dbl)
                    n646 = local read "右180°外全行程间隙"() -> (w1028:dbl)
                    n647 = local read "左180°外全行程间隙"() -> (w1027:dbl)
                    n648 = local read "左180°内全行程间隙"() -> (w1045:dbl)
                    n649 = local read "右最大轴向力(N)"() -> (w1030:dbl)
                    n650 = local read "左轴向力波动(N)"() -> (w1031:dbl)
                    n651 = local read "左最大轴向力(N)"() -> (w1029:dbl)
                    n652 = local read "员工ID"() -> (w1017:string)
                    n653 = local read "右轴向力波动(N)"() -> (w1032:dbl)
                    n654 = Boolean To (0,1)(Boolean=w1038) -> (0, 1=w1040:i16)
                    n655 = local read "中间位置间隙"() -> (w1047:dbl)
                    n656 = local read "总圈数"() -> (w1034:dbl)
                    n657 = local read "总行程"() -> (w1033:dbl)
                    n658 = local read "FGCS"() -> (w1049:string)
                    n659 = local read "KSJJ"() -> (w1051:string)
                    n660 = local read "产品ID"() -> (w1052:string)
                    n661 = Number To Decimal String(number=w1040, width (-)=i16 1 ("宽度(-)")) -> (decimal integer string=w1037:string)
                    n662 = Format Date/Time String(time format string (%c)="%Y%m%d%H%M" ("时间格式字符串(%c)")) -> (date/time string=w1050:string)  [unwired: 2 in]
                    n663 = Number To Fractional String(number=w1033, precision (6)=w1036) -> (F-format string=w1019:string)  [unwired: 2 in]
                    n664 = Number To Fractional String(number=w1028, precision (6)=w1036) -> (F-format string=w1024:string)  [unwired: 2 in]
                    n665 = Number To Fractional String(number=w1031, precision (6)=w1036) -> (F-format string=w1021:string)  [unwired: 2 in]
                    n666 = Number To Fractional String(number=w1035, precision (6)=w1036) -> (F-format string=w1026:string)  [unwired: 2 in]
                    n667 = Number To Fractional String(number=w1030, precision (6)=w1036) -> (F-format string=w1022:string)  [unwired: 2 in]
                    n668 = Number To Fractional String(number=w1032, precision (6)=w1036) -> (F-format string=w1020:string)  [unwired: 2 in]
                    n669 = Number To Fractional String(number=w1045, precision (6)=w1036) -> (F-format string=w1043:string)  [unwired: 2 in]
                    n670 = Number To Fractional String(number=w1029, precision (6)=w1036) -> (F-format string=w1023:string)  [unwired: 2 in]
                    n671 = Number To Fractional String(number=w1034, precision (6)=w1036) -> (F-format string=w1018:string)  [unwired: 2 in]
                    n672 = Number To Fractional String(number=w1027, precision (6)=w1036) -> (F-format string=w1025:string)  [unwired: 2 in]
                    n673 = Number To Fractional String(number=w1047, precision (6)=i16 3 ("精度(6)")) -> (F-format string=w1044:string)  [unwired: 2 in]
                    n674 = Build Array(w1052, w1017, "1", w1037, w1051, w1050, w1049, "Q14073-11A", w1044, w1043, w1026, w1025, w1024, w1023, w1022, w1021, w1020, w1019, w1018) -> (w1042:string[])
                  }
                  frame #2 {
                    n675 = Wait (ms)(milliseconds to wait=u32 500 ("等待时间（毫秒）")) -> ()  [unwired: 1 out]
                    n676 = call "数据库更新.vi"("设备号"="06", "数据"=w1054) -> ()  [unwired: 13 in, 1 out]
                  }
                  frame #3 {
                  }
                }
              }
            }
          }
          frame #9 {
            w1057 = FALSE
            n677 = local write "测头气缸右移"(w1057) -> ()
            n678 = local write "测头气缸左移"(w1057) -> ()
            n679 = local write "产品ID"("") -> ()
            n680 = local write "工步号"(u32 0 ("工步号")) -> ()
          }
        }
      }
    }
    n681 = Wait (ms)(milliseconds to wait=u32 50 ("毫秒倍数")) -> ()  [unwired: 1 out]
    n682 = local read "停止"() -> (w7:bool)
  }
  n683 = while {
    stop <- w1060 stop-if-true
    n684 = event shown="[2] \"参数修改\": 值改变" {
      selector: _ -> [_ _ _ _ _ _]
      dyn-events: _ -> [_ _ _ _ _ _]
      timeout: 500 -> [_ _ _ _ _ _]
      event Timeout {
        n685 = event-data() -> ()  [unwired: 3 out]
      }
      event "停止": Value Change {
        n686 = event-data() -> ()  [unwired: 6 out]
        n687 = flat-sequence {
          frame #0 {
            n688 = Wait (ms)(milliseconds to wait=u32 1000 ("毫秒倍数")) -> ()  [unwired: 1 out]
          }
          frame #1 {
            n689 = Quit LabVIEW(quit? (T)=TRUE ("停止？(T)")) -> ()
          }
        }
      }
      event "参数修改": Value Change {
        n690 = event-data() -> ()  [unwired: 6 out]
        n691 = while {
          i -> [w1067]
          stop <- w1066 stop-if-true
          n692 = local read "参数浏览表"() -> (w1069:string[][])
          n693 = local read "型号数量"() -> (w1068:i32)
          n694 = Wait Until Next ms Multiple(millisecond multiple=u32 50 ("毫秒倍数")) -> ()  [unwired: 1 out]
          n695 = Greater Or Equal?(x=w1067, y=w1068) -> (x >= y?=w1066:bool)
          n696 = Index Array(array=w1069, index (col)=w1067) -> (element=w1065:string[])  [unwired: 1 in]
          n697 = stacked-sequence {
            tunnel: w1065 -> [w1111]
            frame #0 {
              n698 = Index Array(array=w1111, index #1=0 ("索引"), index #2=2 ("索引"), index #3=3 ("索引"), index #4=4 ("索引"), index #5=5 ("索引"), index #6=6 ("索引"), index #7=7 ("索引"), index #8=8 ("索引"), index #9=9 ("索引"), index #10=10 ("索引"), index #11=11 ("索引"), index #12=12 ("索引"), index #13=13 ("索引"), index #14=14 ("索引"), index #15=15 ("索引"), index #16=16 ("索引"), index #17=17 ("索引"), index #18=18 ("索引"), index #19=19 ("索引"), index #20=20 ("索引"), index #21=21 ("索引"), index #22=22 ("索引"), index #23=23 ("索引")) -> (element #1=w1071:string, element #2=w1107:string, element #3=w1106:string, element #4=w1105:string, element #5=w1104:string, element #6=w1103:string, element #7=w1102:string, element #8=w1101:string, element #9=w1100:string, element #10=w1099:string, element #11=w1098:string, element #12=w1089:string, element #13=w1088:string, element #14=w1087:string, element #15=w1086:string, element #16=w1085:string, element #17=w1084:string, element #18=w1081:string, element #19=w1080:string, element #20=w1078:string, element #21=w1077:string, element #22=w1076:string, element #23=w1075:string)
              n699 = call "创建文本"("测头机构轴移动速度"=w1107, "测头机构轴检测位"=w1106, "测头机构轴待检位"=w1105, "测头机构轴后退位"=w1104, "齿条移动速度"=w1103, "齿条左极限"=w1102, "齿条右极限"=w1101, "旋转齿条轴找帽转速"=w1100, "旋转齿条轴测量转速"=w1099, "测量点扭矩"=w1098, "总行程最小值"=w1089, "总行程最大值"=w1088, "最大轴向力"=w1087, "轴向力波动"=w1086, "平均轴向力最小值"=w1085, "平均轴向力最大值"=w1084, "总圈数最小值"=w1081, "总圈数最大值"=w1080, "中间位置"=w1078, "中间间隙标准"=w1077, "180内间隙标准"=w1076, "180外间隙标准"=w1075, "产品型号"=w1071) -> ("Result"=w1097:string)  [unwired: 3 in, 1 out]
              n700 = local read "ADODB._Connection Out 2"() -> (w1096:refnum<k7>)
              n701 = call "SQL Execute.vi"("Command Text"=w1097, "ADODB._Connection In"=w1096) -> ("error out"=w1109:errorcluster, "ADODB._Connection Out"=w1110:refnum<k7>)  [unwired: 6 in, 2 out]
              n702 = call "ADO Connection Close.vi"("error in (no error)"=w1109, "ADODB._Connection In"=w1110) -> ("error out"=→"error out":errorcluster)  [unwired: 8 in, 1 out]
            }
          }
        }
      }
      event "参数查询": Value Change {
        n703 = event-data() -> ()  [unwired: 6 out]
        n704 = flat-sequence {
          tunnel: [w1134] -> w1127
          tunnel: [w1133] -> w1126
          tunnel: [w1132] -> w1123
          tunnel: w1127 -> [w1138]
          tunnel: w1126 -> [w1140]
          tunnel: [w1140] -> w1125
          tunnel: [w1139] -> w1124
          tunnel: w1123 -> [w1139]
          tunnel: w1125 -> [_]
          tunnel: w1124 -> [_]
          frame #0 {
            n705 = call-poly <vilib>:"Read From Spreadsheet File.vi"("file path (dialog if empty)"=path "D:/Q14070-Z060人机界面/参数/参数项.txt") -> ("first row"=w1128:string[])  [unwired: 6 in, 4 out]
            n706 = property on="参数浏览表" class="Tbl (严格)"("Row Headers[]"=w1128) -> ()  [unwired: 2 in, 2 out]
          }
          frame #1 {
            n707 = local read "ADODB._Connection Out 2"() -> (w1131:refnum<k7>)
            n708 = call "SQL Execute.vi"("Command Text"="SELECT * FROM 测试参数表;", "ADODB._Connection In"=w1131) -> ("error out"=w1132:errorcluster, "Data"=w1136:string[][], "ADODB._Connection Out"=w1133:refnum<k7>)  [unwired: 6 in, 1 out]
            n709 = Transpose 2D Array "二维数组转置"(2D array=w1136) -> (transposed array=w1134:string[][])
            n710 = Index Array(array=w1134, index (row)=0 ("索引 (行)")) -> (element=w1135:string[])  [unwired: 1 in]
            n711 = property on="参数浏览表" class="Tbl (严格)"("Column Headers[]"=w1135) -> ()  [unwired: 2 in, 2 out]
          }
          frame #2 {
            n712 = local write "参数浏览表"(w1138) -> ()
          }
          frame #3 {
          }
        }
      }
      event "传感器参数保存": Value Change {
        n713 = event-data() -> ()  [unwired: 6 out]
        n714 = flat-sequence {
          frame #0 {
            n715 = local read "齿条推拉力零点偏移"() -> (w1145:dbl)
            n716 = local read "齿条推拉力比例偏移"() -> (w1141:dbl)
            n717 = local read "间隙位移零点偏移"() -> (w1152:dbl)
            n718 = local read "齿条扭矩零点偏移"() -> (w1144:dbl)
            n719 = local read "间隙位移比例偏移"() -> (w1142:dbl)
            n720 = local read "齿条扭矩比例偏移"() -> (w1143:dbl)
            n721 = local read "ADODB._Connection Out 2"() -> (w1160:refnum<k7>)
            n722 = Number To Fractional String(number=w1152, precision (6)=i16 2 ("精度(6)")) -> (F-format string=w1159:string)  [unwired: 2 in]
            n723 = Number To Fractional String(number=w1145, precision (6)=i16 2 ("精度(6)")) -> (F-format string=w1158:string)  [unwired: 2 in]
            n724 = Number To Fractional String(number=w1144, precision (6)=i16 2 ("精度(6)")) -> (F-format string=w1157:string)  [unwired: 2 in]
            n725 = Number To Fractional String(number=w1142, precision (6)=i16 2 ("精度(6)")) -> (F-format string=w1156:string)  [unwired: 2 in]
            n726 = Number To Fractional String(number=w1141, precision (6)=i16 2 ("精度(6)")) -> (F-format string=w1155:string)  [unwired: 2 in]
            n727 = Number To Fractional String(number=w1143, precision (6)=i16 2 ("精度(6)")) -> (F-format string=w1154:string)  [unwired: 2 in]
            n728 = call "创建文本3"("4"=w1156, "6"=w1154, "1"=w1159, "2"=w1158, "3"=w1157, "5"=w1155) -> ("Result"=w1161:string)  [unwired: 8 in, 1 out]
            n729 = call "SQL Execute.vi"("Command Text"=w1161, "ADODB._Connection In"=w1160) -> ("error out"=→"error out 4":errorcluster)  [unwired: 6 in, 3 out]
          }
        }
      }
      event "产品ID": Value Change {
        n730 = event-data() -> ()  [unwired: 7 out]
        n731 = Format Date/Time String(time format string (%c)="%Y%m%d%H%M" ("时间格式字符串(%c)")) -> (date/time string=w1162:string)  [unwired: 2 in]
        n732 = local write "KSJJ"(w1162) -> ()
      }
    }
    n733 = Wait (ms)(milliseconds to wait=u32 50 ("毫秒倍数")) -> ()  [unwired: 1 out]
    n734 = local read "停止"() -> (w1060:bool)
  }
  n735 = disable-structure shown="禁用" {
    frame Disabled {
      n736 = flat-sequence {
        frame #0 {
          n737 = local read "中间位置最大间隙标准(mm)"() -> (w1165:dbl)
          n738 = local read "中间位置间隙"() -> (w1166:dbl)
          n739 = local read "最小间隙(mm)"() -> (w1164:dbl)
          n740 = In Range and Coerce(upper limit=w1165, x=w1166, lower limit=w1164) -> (In Range?=w1169:bool)  [unwired: 1 out]
          n741 = case shown="假" w1169 {
            tunnel: [FALSE ("本序合格") TRUE ("本序合格")] -> w1168
            tunnel: [w1174 0.0 ("需调整角度(度)")] -> w1167
            tunnel: w1166 -> [w1172 _]
            tunnel: w1165 -> [w1171 _]
            tunnel: w1164 -> [w1170 _]
            frame False {
              n742 = xnode "公式"("X"=w1172, "Xmax"=w1171, "Xmin"=w1170) -> ("结果"=w1174:dbl)  [unwired: 1 in, 1 out]
            }
            frame True {
            }
          }
          n743 = local write "单点间隙合格"(w1168) -> ()
          n744 = local write "需调整角度(度)"(w1167) -> ()
        }
      }
    }
    frame Enabled {
    }
  }
  n745 = while {
    stop <- w1190 stop-if-true
    n746 = stacked-sequence {
      frame #0 {
        n747 = flat-sequence {
          frame #0 {
          }
          frame #1 {
            "PLC" <- "阻挡"
          }
          frame #2 {
            n748 = First Call?() -> (First Call?: T/F=w1192:bool)
            n749 = case shown="真" w1192 {
              frame False {
              }
              frame True {
                n750 = call "员工管理测试程序.vi"() -> ("员工姓名"=w1194:string, "员工ID"=w1193:string)  [unwired: 10 in]
                n751 = local write "员工ID"(w1193) -> ()
                n752 = local write "员工姓名"(w1194) -> ()
              }
            }
          }
          frame #3 {
          }
          frame #4 {
          }
          frame #5 {
          }
          frame #6 {
          }
        }
      }
      frame #1 {
        n753 = flat-sequence {
          frame #0 {
            n754 = property on="型号选择" class="Ring (严格)"() -> ("RingText.Text"=w1198:string)  [unwired: 2 in, 2 out]
            n755 = case shown="\"J728\"" w1198 {
              frame "J709", Default {
                w1199 = FALSE ("可见")
                w1200 = TRUE ("可见")
                n756 = property on="右180°内全行程间隙" class="DigNum (严格)"("Visible"=w1199) -> ()  [unwired: 2 in, 2 out]
                n757 = property on="右180°外全行程间隙" class="DigNum (严格)"("Visible"=w1199) -> ()  [unwired: 2 in, 2 out]
                n758 = property on="左180°外全行程间隙" class="DigNum (严格)"("Visible"=w1199) -> ()  [unwired: 2 in, 2 out]
                n759 = property on="左180°内全行程间隙" class="DigNum (严格)"("Visible"=w1199) -> ()  [unwired: 2 in, 2 out]
                n760 = property on="右全行程间隙" class="DigNum (严格)"("Visible"=w1200) -> ()  [unwired: 2 in, 2 out]
                n761 = property on="左全行程间隙" class="DigNum (严格)"("Visible"=w1200) -> ()  [unwired: 2 in, 2 out]
              }
              frame "J706" {
                w1201 = TRUE ("可见")
                w1202 = FALSE ("可见")
                n762 = property on="右180°内全行程间隙" class="DigNum (严格)"("Visible"=w1201) -> ()  [unwired: 2 in, 2 out]
                n763 = property on="右180°外全行程间隙" class="DigNum (严格)"("Visible"=w1201) -> ()  [unwired: 2 in, 2 out]
                n764 = property on="左180°外全行程间隙" class="DigNum (严格)"("Visible"=w1201) -> ()  [unwired: 2 in, 2 out]
                n765 = property on="左180°内全行程间隙" class="DigNum (严格)"("Visible"=w1201) -> ()  [unwired: 2 in, 2 out]
                n766 = property on="右全行程间隙" class="DigNum (严格)"("Visible"=w1202) -> ()  [unwired: 2 in, 2 out]
                n767 = property on="左全行程间隙" class="DigNum (严格)"("Visible"=w1202) -> ()  [unwired: 2 in, 2 out]
              }
              frame "J728" {
                w1203 = TRUE ("可见")
                w1204 = FALSE ("可见")
                n768 = property on="右180°内全行程间隙" class="DigNum (严格)"("Visible"=w1203) -> ()  [unwired: 2 in, 2 out]
                n769 = property on="右180°外全行程间隙" class="DigNum (严格)"("Visible"=w1203) -> ()  [unwired: 2 in, 2 out]
                n770 = property on="左180°外全行程间隙" class="DigNum (严格)"("Visible"=w1203) -> ()  [unwired: 2 in, 2 out]
                n771 = property on="左180°内全行程间隙" class="DigNum (严格)"("Visible"=w1203) -> ()  [unwired: 2 in, 2 out]
                n772 = property on="右全行程间隙" class="DigNum (严格)"("Visible"=w1204) -> ()  [unwired: 2 in, 2 out]
                n773 = property on="左全行程间隙" class="DigNum (严格)"("Visible"=w1204) -> ()  [unwired: 2 in, 2 out]
              }
            }
          }
          frame #1 {
            (unwired) string[] ["I急停按钮", "I自动旋钮", "I启动按钮", "I备用按钮", "I复位按钮", "I上阻挡器放行", "I下阻挡器放行", "I进支线按钮"] ("I0说明")
            (unwired) string[] ["I出支线按钮", "I主线顶升按钮", "I主线下降按钮", "I支线顶升按钮", "I支线下降按钮", "I气压报警", "未使用", "未使用"] ("I0说明")
            n774 = local read "间隙位移(mm)"() -> (w1207:dbl)
            n775 = Greater Or Equal?(x=w1207, y=4.0) -> (x >= y?=w1205:bool)
            n776 = case shown="真" w1205 {
              frame False {
              }
              frame True {
                n777 = local write "测头机构轴使能"(FALSE ("测头机构轴使能")) -> ()
              }
            }
          }
          frame #2 {
            (unwired) string[] ["I电动缸SRDY", "I电动缸ZSPD", "I电动缸ALRM", "I间隙进给SRDY", "I间隙进给ZSPD", "I间隙进给ALRM", "I间隙旋转SRPD", "I间隙旋转ZSPD"] ("I0说明")
            n778 = local read "测头机构轴位置(mm)"() -> (w1211:dbl)
            n779 = Greater Or Equal?(x=w1211, y=90.0) -> (x >= y?=w1209:bool)
            n780 = case shown="假" w1209 {
              frame False {
                w1212 = T5."Enabled" ("禁用")
                n781 = property on="测头气缸右移" class="Bool"("DisabledEnum"=w1212) -> ()  [unwired: 2 in, 2 out]
                n782 = property on="测头气缸左移" class="Bool"("DisabledEnum"=w1212) -> ()  [unwired: 2 in, 2 out]
                n783 = property on="测头气缸右移" class="Bool (严格)"("DisabledEnum"=w1212) -> ()  [unwired: 2 in, 2 out]
                n784 = property on="测头气缸左移" class="Bool (严格)"("DisabledEnum"=w1212) -> ()  [unwired: 2 in, 2 out]
              }
              frame True {
                w1213 = T5."Disabled" ("禁用")
                w1214 = FALSE ("测头气缸右移")
                n785 = local write "测头气缸右移"(w1214) -> ()
                n786 = local write "测头气缸左移"(w1214) -> ()
                n787 = property on="测头气缸右移" class="Bool"("DisabledEnum"=w1213) -> ()  [unwired: 2 in, 2 out]
                n788 = property on="测头气缸左移" class="Bool"("DisabledEnum"=w1213) -> ()  [unwired: 2 in, 2 out]
                n789 = property on="测头气缸右移" class="Bool (严格)"("DisabledEnum"=w1213) -> ()  [unwired: 2 in, 2 out]
                n790 = property on="测头气缸左移" class="Bool (严格)"("DisabledEnum"=w1213) -> ()  [unwired: 2 in, 2 out]
              }
            }
          }
          frame #3 {
            (unwired) string[] ["I间隙旋转ALRM", "I扭矩旋转SRPD", "I扭矩旋转ZSPD", "I扭矩旋转ALRM", "I拧紧机合格", "I拧紧机不合格", "I拧紧机报警", "未使用"] ("I0说明")
          }
        }
        n791 = local read "急停"() -> (w1197:bool)
        n792 = local read "复位"() -> (w1196:bool)
        n793 = Compound Arithmetic op=OR(invert w1197, w1196) -> (→"循环退出":bool)
      }
      frame #2 {
        n794 = flat-sequence {
          frame #0 {
            (unwired) string[] ["I自制气缸进位", "I自制气缸原位", "I上工位检测", "I本工位检测", "I下工位检测", "I主线顶升上位", "I主线顶升下位", "I支线顶升上位"] ("I0说明")
          }
          frame #1 {
            (unwired) string[] ["I支线顶升下位", "I支线进到位", "I支线退到位", "I位移气缸原位", "I位移气缸进位", "I拧紧机在位", "I电动缸原位", "I电动缸进位"] ("I0说明")
          }
          frame #2 {
            (unwired) string[] ["未使用", "未使用", "未使用", "未使用", "未使用", "未使用", "未使用", "未使用"] ("I0说明")
          }
          frame #3 {
            (unwired) string[] ["未使用", "未使用", "未使用", "未使用", "未使用", "未使用", "未使用", "未使用"] ("I0说明")
          }
        }
        n795 = local read "本测试状态"() -> (w1216:bool)
        n796 = local read "本自动状态"() -> (w1217:bool)
        n797 = local read "本备料状态"() -> (w1215:bool)
        n798 = local write "本测试状态H"(w1216) -> ()
        n799 = local write "本自动状态H"(w1217) -> ()
        n800 = local write "本备料状态H"(w1215) -> ()
      }
      frame #3 {
        n801 = local read "报警工步号"() -> (w1219:dbl)
        n802 = local read "工步号"() -> (w1221:u32)
        n803 = case shown="0, 默认" w1221 {
          tunnel: [w1231 "请取胶瓶" ("工步描述") "请对锁紧螺母加力" ("工步描述") "灵敏度测试中" ("工步描述") "有油刚度测试中" ("工步描述") "安装好锁紧螺母后，按顶升按钮，夹具夹紧" ("工步描述") "请点击启动按钮进行试验" ("工步描述") "探头气缸右移" ("工步描述") "电动缸前进找中" ("工步描述") "探头前进测试开始" ("工步描述") "探头退回" ("工步描述") "轴向力测试中" ("工步描述") "测头后退夹抓松开" ("工步描述") "伺服回零" ("工步描述") "力特性试验完成" ("工步描述") "套好输出轴把手，按启动按钮，做回正力试验" ("工步描述") "回正力试验中" ("工步描述") "试验完成，将把手拉回，取下油管，按顶升按钮" ("工步描述") "拆下锁紧螺母和输入轴万向节，按顶升按钮" ("工步描述")] -> w1220
          frame 0, Default {
            n804 = local read "联线按钮"() -> (w1230:bool)
            n805 = case shown="真" w1230 {
              tunnel: ["等待工件" ("工步描述") "等待扫描条码" ("工步描述")] -> w1231
              frame False {
              }
              frame True {
              }
            }
          }
          frame 1 {
          }
          frame 2 {
          }
          frame 3 {
          }
          frame 4 {
          }
          frame 5 {
          }
          frame 6 {
          }
          frame 10 {
          }
          frame 15 {
          }
          frame 20 {
          }
          frame 30 {
          }
          frame 40 {
          }
          frame 45 {
          }
          frame 50 {
          }
          frame 55 {
          }
          frame 60 {
          }
          frame 70 {
          }
          frame 80 {
          }
          frame 56 {
          }
        }
        "工步提示" <- w1220
        n806 = case shown="3" w1219 {
          tunnel: [_ "操作步骤错请取胶瓶" "操作步骤错误请点标" "测头气缸不在原位" "急停被按下" "气压报警" "电动缸伺服报警" "旋转伺服服报警" "测头伺服服报警"] -> w1218
          frame 0, Default {
          }
          frame 1 {
          }
          frame 3 {
          }
          frame 2 {
          }
          frame 4 {
          }
          frame 5 {
          }
          frame 6 {
          }
          frame 7 {
          }
          frame 8 {
          }
        }
        "报警提示" <- w1218
      }
      frame #4 {
        n807 = local read "急停"() -> (w1253:bool)
        n808 = local read "红灯"() -> (w1252:bool)
        n809 = local read "复位"() -> (w1255:bool)
        n810 = local read "红灯"() -> (w1254:bool)
        n811 = case shown="假" w1253 {
          frame False {
            n812 = local write "红灯"(TRUE ("红灯")) -> ()
          }
          frame True {
            n813 = local write "红灯"(FALSE ("复位")) -> ()
          }
        }
        n814 = case shown="真" w1252 {
          frame False {
          }
          frame True {
            n815 = local write "回零完成"(FALSE ("夹头夹紧控制")) -> ()
          }
        }
        n816 = local read "停止"() -> (w1257:bool)
        n817 = Compound Arithmetic op=OR(w1255, w1257, w1254) -> (w1256:bool)
        n818 = case shown="真" w1256 {
          frame False {
          }
          frame True {
            n819 = local read "测头机构电机"() -> (w1261:u32)
            n820 = local read "旋转齿条电机"() -> (w1262:u32)
            n821 = local read "电动缸电机"() -> (w1263:u32)
            n822 = call "PCI1220U停止.vi"("AxisHandle IN"=w1262) -> ()  [unwired: 9 in, 2 out]
            n823 = call "PCI1220U停止.vi"("AxisHandle IN"=w1263) -> ()  [unwired: 9 in, 2 out]
            n824 = call "PCI1220U停止.vi"("AxisHandle IN"=w1261) -> ()  [unwired: 9 in, 2 out]
          }
        }
      }
      frame #5 {
        n825 = local read "齿条扭矩(Nm)"() -> (w1266:dbl)
        n826 = local read "黄灯"() -> (w1264:bool)
        n827 = local read "旋转齿条轴左转"() -> (w1272:bool)
        n828 = Absolute Value(x=w1266) -> (abs(x)=w1271:dbl)
        n829 = local read "旋转齿条轴右转"() -> (w1267:bool)
        n830 = Not(x=w1272) -> (.not. x?=w1268:bool)
        n831 = Less?(x=w1271, y=20.0) -> (x < y?=w1269:bool)
        n832 = Compound Arithmetic op=AND(w1267, w1268, w1269, w1264) -> (w1265:bool)
        n833 = case shown="真" w1265 {
          frame False {
          }
          frame True {
            n834 = flat-sequence {
              tunnel: [w1276] -> w1274
              tunnel: w1274 -> [w1278]
              tunnel: [w1278] -> w1273
              tunnel: w1273 -> [w1289]
              frame #0 {
                n835 = local read "旋转齿条电机"() -> (w1275:u32)
                n836 = call "PCI1220U运行.vi"("方向"=enum32{"Negative", "Positive"}."Negative" ("Direction"), "AxisHandle IN"=w1275) -> ("AxisHandle OUT"=w1276:u32)  [unwired: 9 in]
              }
              frame #1 {
                n837 = while {
                  stop <- w1282 stop-if-true
                  n838 = Wait (ms)(milliseconds to wait=u32 50 ("毫秒倍数")) -> ()  [unwired: 1 out]
                  n839 = local read "齿条扭矩(Nm)"() -> (w1287:dbl)
                  n840 = local read "旋转齿条轴右转"() -> (w1284:bool)
                  n841 = local read "红灯"() -> (w1279:bool)
                  n842 = local read "复位"() -> (w1280:bool)
                  n843 = Absolute Value(x=w1287) -> (abs(x)=w1286:dbl)
                  n844 = Not(x=w1284) -> (.not. x?=w1281:bool)
                  n845 = Greater?(x=w1286, y=10.0) -> (0:w1283:bool)
                  n846 = Compound Arithmetic op=OR(w1283, w1281, w1280, w1279) -> (w1282:bool)
                }
              }
              frame #2 {
                n847 = call "PCI1220U停止.vi"("AxisHandle IN"=w1289) -> ()  [unwired: 9 in, 2 out]
              }
            }
          }
        }
      }
      frame #6 {
        n848 = local read "齿条扭矩(Nm)"() -> (w1294:dbl)
        n849 = local read "旋转齿条轴右转"() -> (w1298:bool)
        n850 = Absolute Value(x=w1294) -> (abs(x)=w1293:dbl)
        n851 = local read "旋转齿条轴左转"() -> (w1296:bool)
        n852 = local read "黄灯"() -> (w1290:bool)
        n853 = Not(x=w1298) -> (.not. x?=w1295:bool)
        n854 = Less?(x=w1293, y=20.0) -> (x < y?=w1291:bool)
        n855 = Compound Arithmetic op=AND(w1296, w1295, w1291, w1290) -> (w1297:bool)
        n856 = case shown="真" w1297 {
          frame False {
          }
          frame True {
            n857 = flat-sequence {
              tunnel: [w1302] -> w1300
              tunnel: w1300 -> [w1304]
              tunnel: [w1304] -> w1299
              tunnel: w1299 -> [w1315]
              frame #0 {
                n858 = local read "旋转齿条电机"() -> (w1301:u32)
                n859 = call "PCI1220U运行.vi"("方向"=enum32{"Negative", "Positive"}."Positive" ("Direction"), "AxisHandle IN"=w1301) -> ("AxisHandle OUT"=w1302:u32)  [unwired: 9 in]
              }
              frame #1 {
                n860 = while {
                  stop <- w1307 stop-if-true
                  n861 = Wait (ms)(milliseconds to wait=u32 50 ("毫秒倍数")) -> ()  [unwired: 1 out]
                  n862 = local read "齿条扭矩(Nm)"() -> (w1313:dbl)
                  n863 = local read "旋转齿条轴左转"() -> (w1310:bool)
                  n864 = local read "红灯"() -> (w1305:bool)
                  n865 = local read "复位"() -> (w1306:bool)
                  n866 = Absolute Value(x=w1313) -> (abs(x)=w1312:dbl)
                  n867 = Not(x=w1310) -> (.not. x?=w1308:bool)
                  n868 = Greater?(x=w1312, y=10.0) -> (0:w1309:bool)
                  n869 = Compound Arithmetic op=OR(w1306, w1305, w1309, w1308) -> (w1307:bool)
                }
              }
              frame #2 {
                n870 = call "PCI1220U停止.vi"("AxisHandle IN"=w1315) -> ()  [unwired: 9 in, 2 out]
              }
            }
          }
        }
      }
      frame #7 {
        n871 = local read "齿条推拉力(N)"() -> (w1320:dbl)
        n872 = local read "电动缸前进"() -> (w1317:bool)
        n873 = local read "电动缸后退"() -> (w1316:bool)
        n874 = Absolute Value(x=w1320) -> (abs(x)=w1324:dbl)
        n875 = local read "黄灯"() -> (w1318:bool)
        n876 = Not(x=w1316) -> (.not. x?=w1321:bool)
        n877 = Less?(x=w1324, y=1000.0) -> (x < y?=w1322:bool)
        n878 = Compound Arithmetic op=AND(w1317, w1321, w1318, w1322) -> (w1319:bool)
        n879 = case shown="真" w1319 {
          frame False {
          }
          frame True {
            n880 = flat-sequence {
              tunnel: [w1328] -> w1326
              tunnel: w1326 -> [w1330]
              tunnel: [w1330] -> w1325
              tunnel: w1325 -> [w1341]
              frame #0 {
                n881 = local read "电动缸电机"() -> (w1327:u32)
                n882 = call "PCI1220U运行.vi"("方向"=enum32{"Negative", "Positive"}."Positive" ("Direction"), "AxisHandle IN"=w1327) -> ("AxisHandle OUT"=w1328:u32)  [unwired: 9 in]
              }
              frame #1 {
                n883 = while {
                  stop <- w1338 stop-if-true
                  n884 = local read "电动缸前进"() -> (w1335:bool)
                  n885 = local read "齿条推拉力(N)"() -> (w1332:dbl)
                  n886 = Wait (ms)(milliseconds to wait=u32 50 ("毫秒倍数")) -> ()  [unwired: 1 out]
                  n887 = Absolute Value(x=w1332) -> (abs(x)=w1334:dbl)
                  n888 = local read "红灯"() -> (w1336:bool)
                  n889 = local read "复位"() -> (w1337:bool)
                  n890 = Greater?(x=w1334, y=1000.0) -> (0:w1331:bool)
                  n891 = Not(x=w1335) -> (.not. x?=w1339:bool)
                  n892 = Compound Arithmetic op=OR(w1337, w1336, w1339, w1331) -> (w1338:bool)
                }
              }
              frame #2 {
                n893 = call "PCI1220U停止.vi"("AxisHandle IN"=w1341) -> ()  [unwired: 9 in, 2 out]
              }
            }
          }
        }
      }
      frame #8 {
        n894 = local read "电动缸前进"() -> (w1342:bool)
        n895 = local read "齿条推拉力(N)"() -> (w1346:dbl)
        n896 = local read "电动缸后退"() -> (w1343:bool)
        n897 = Absolute Value(x=w1346) -> (abs(x)=w1350:dbl)
        n898 = local read "黄灯"() -> (w1344:bool)
        n899 = Not(x=w1342) -> (.not. x?=w1347:bool)
        n900 = Less?(x=w1350, y=1000.0) -> (x < y?=w1348:bool)
        n901 = Compound Arithmetic op=AND(w1343, w1347, w1344, w1348) -> (w1345:bool)
        n902 = case shown="真" w1345 {
          frame False {
          }
          frame True {
            n903 = flat-sequence {
              tunnel: [w1354] -> w1352
              tunnel: w1352 -> [w1356]
              tunnel: [w1356] -> w1351
              tunnel: w1351 -> [w1367]
              frame #0 {
                n904 = local read "电动缸电机"() -> (w1353:u32)
                n905 = call "PCI1220U运行.vi"("方向"=enum32{"Negative", "Positive"}."Negative" ("Direction"), "AxisHandle IN"=w1353) -> ("AxisHandle OUT"=w1354:u32)  [unwired: 9 in]
              }
              frame #1 {
                n906 = while {
                  stop <- w1364 stop-if-true
                  n907 = local read "电动缸后退"() -> (w1361:bool)
                  n908 = local read "齿条推拉力(N)"() -> (w1360:dbl)
                  n909 = Wait (ms)(milliseconds to wait=u32 50 ("毫秒倍数")) -> ()  [unwired: 1 out]
                  n910 = Absolute Value(x=w1360) -> (abs(x)=w1358:dbl)
                  n911 = local read "红灯"() -> (w1363:bool)
                  n912 = local read "复位"() -> (w1362:bool)
                  n913 = Greater?(x=w1358, y=1000.0) -> (0:w1357:bool)
                  n914 = Not(x=w1361) -> (.not. x?=w1365:bool)
                  n915 = Compound Arithmetic op=OR(w1362, w1363, w1365, w1357) -> (w1364:bool)
                }
              }
              frame #2 {
                n916 = call "PCI1220U停止.vi"("AxisHandle IN"=w1367) -> ()  [unwired: 9 in, 2 out]
              }
            }
          }
        }
      }
      frame #9 {
        n917 = local read "测头机构轴后退"() -> (w1368:bool)
        n918 = local read "测头机构轴前进"() -> (w1369:bool)
        n919 = local read "黄灯"() -> (w1370:bool)
        n920 = Not(x=w1368) -> (.not. x?=w1372:bool)
        n921 = Compound Arithmetic op=AND(w1369, w1372, w1370) -> (w1371:bool)
        n922 = case shown="真" w1371 {
          frame False {
          }
          frame True {
            n923 = flat-sequence {
              tunnel: [w1376] -> w1374
              tunnel: w1374 -> [w1378]
              tunnel: [w1378] -> w1373
              tunnel: w1373 -> [w1385]
              frame #0 {
                n924 = local read "测头机构电机"() -> (w1375:u32)
                n925 = call "PCI1220U运行.vi"("方向"=enum32{"Negative", "Positive"}."Positive" ("Direction"), "AxisHandle IN"=w1375) -> ("AxisHandle OUT"=w1376:u32)  [unwired: 9 in]
              }
              frame #1 {
                n926 = while {
                  stop <- w1382 stop-if-true
                  n927 = local read "测头机构轴前进"() -> (w1379:bool)
                  n928 = Wait (ms)(milliseconds to wait=u32 50 ("毫秒倍数")) -> ()  [unwired: 1 out]
                  n929 = local read "红灯"() -> (w1380:bool)
                  n930 = local read "复位"() -> (w1381:bool)
                  n931 = Not(x=w1379) -> (.not. x?=w1383:bool)
                  n932 = Compound Arithmetic op=OR(w1381, w1380, w1383) -> (w1382:bool)
                }
              }
              frame #2 {
                n933 = call "PCI1220U停止.vi"("AxisHandle IN"=w1385) -> ()  [unwired: 9 in, 2 out]
              }
            }
          }
        }
      }
      frame #10 {
        n934 = local read "测头机构轴前进"() -> (w1386:bool)
        n935 = local read "测头机构轴后退"() -> (w1387:bool)
        n936 = local read "黄灯"() -> (w1388:bool)
        n937 = Not(x=w1386) -> (.not. x?=w1390:bool)
        n938 = Compound Arithmetic op=AND(w1387, w1390, w1388) -> (w1389:bool)
        n939 = case shown="真" w1389 {
          frame False {
          }
          frame True {
            n940 = flat-sequence {
              tunnel: [w1394] -> w1392
              tunnel: w1392 -> [w1396]
              tunnel: [w1396] -> w1391
              tunnel: w1391 -> [w1403]
              frame #0 {
                n941 = local read "测头机构电机"() -> (w1393:u32)
                n942 = call "PCI1220U运行.vi"("方向"=enum32{"Negative", "Positive"}."Negative" ("Direction"), "AxisHandle IN"=w1393) -> ("AxisHandle OUT"=w1394:u32)  [unwired: 9 in]
              }
              frame #1 {
                n943 = while {
                  stop <- w1400 stop-if-true
                  n944 = local read "测头机构轴后退"() -> (w1397:bool)
                  n945 = Wait (ms)(milliseconds to wait=u32 50 ("毫秒倍数")) -> ()  [unwired: 1 out]
                  n946 = local read "红灯"() -> (w1399:bool)
                  n947 = local read "复位"() -> (w1398:bool)
                  n948 = Not(x=w1397) -> (.not. x?=w1401:bool)
                  n949 = Compound Arithmetic op=OR(w1398, w1399, w1401) -> (w1400:bool)
                }
              }
              frame #2 {
                n950 = call "PCI1220U停止.vi"("AxisHandle IN"=w1403) -> ()  [unwired: 9 in, 2 out]
              }
            }
          }
        }
      }
      frame #11 {
        n951 = local read "电动缸回零"() -> (w1404:bool)
        n952 = case shown="真" w1404 {
          frame False {
          }
          frame True {
            n953 = stacked-sequence {
              frame #0 {
                n954 = flat-sequence {
                  tunnel: [w1420] -> w1410
                  tunnel: [w1413] -> w1409
                  tunnel: w1410 -> [w1423]
                  tunnel: [w1423] -> w1408
                  tunnel: [w1421] -> w1407
                  tunnel: w1409 -> [w1421]
                  tunnel: w1408 -> [w1425]
                  tunnel: [w1425] -> w1406
                  tunnel: w1407 -> [w1424]
                  tunnel: [w1424] -> w1405
                  tunnel: w1406 -> [w1441]
                  tunnel: w1405 -> [w1440]
                  frame #0 {
                    n955 = local write "电动缸速度(mm/s)"(15.0 ("电动缸速度(mm/s)")) -> ()
                    n956 = local write "测头机构轴速度(mm/s)"(10.0 ("电动缸速度(mm/s)")) -> ()
                  }
                  frame #1 {
                    n957 = local read "测头机构电机"() -> (w1417:u32)
                    n958 = local read "电动缸电机"() -> (w1414:u32)
                    n959 = call <userlib>:"Acm_AxHome.vi"("DirMode"=u32 1, "HomeMode"=u32 11, "AxisHandle"=w1414) -> ("AxisHandle"=w1413:u32)  [unwired: 1 in, 2 out]
                    n960 = call <userlib>:"Acm_AxHome.vi"("DirMode"=u32 0, "HomeMode"=u32 11, "AxisHandle"=w1417) -> ("AxisHandle"=w1420:u32)  [unwired: 1 in, 2 out]
                  }
                  frame #2 {
                    n961 = Wait Until Next ms Multiple(millisecond multiple=u32 100 ("毫秒倍数")) -> ()  [unwired: 1 out]
                  }
                  frame #3 {
                    n962 = while {
                      tunnel: w1424 -> [w1432]
                      stop <- w1427 stop-if-true
                      n963 = call <userlib>:"Acm_AxGetCmdVelocity.vi"("AxisHandle"=w1432) -> ("Velocity"=w1431:dbl)  [unwired: 1 in, 3 out]
                      n964 = Wait Until Next ms Multiple(millisecond multiple=u32 50 ("毫秒倍数")) -> ()  [unwired: 1 out]
                      n965 = Equal To 0?(x=w1431) -> (x = 0?=w1426:bool)
                      n966 = local read "急停"() -> (w1428:bool)
                      n967 = local read "复位"() -> (w1429:bool)
                      n968 = Compound Arithmetic op=OR(invert w1428, w1429, w1426) -> (w1427:bool)
                    }
                    n969 = while {
                      tunnel: w1425 -> [w1439]
                      stop <- w1435 stop-if-true
                      n970 = call <userlib>:"Acm_AxGetCmdVelocity.vi"("AxisHandle"=w1439) -> ("Velocity"=w1438:dbl)  [unwired: 1 in, 3 out]
                      n971 = Wait Until Next ms Multiple(millisecond multiple=u32 50 ("毫秒倍数")) -> ()  [unwired: 1 out]
                      n972 = Equal To 0?(x=w1438) -> (x = 0?=w1436:bool)
                      n973 = local read "急停"() -> (w1433:bool)
                      n974 = local read "复位"() -> (w1434:bool)
                      n975 = Compound Arithmetic op=OR(invert w1433, w1434, w1436) -> (w1435:bool)
                    }
                  }
                  frame #4 {
                    n976 = call "PCI1220U角度置零.vi"("AxisHandle IN"=w1440) -> ()  [unwired: 10 in, 1 out]
                    n977 = call "PCI1220U角度置零.vi"("AxisHandle IN"=w1441) -> ()  [unwired: 10 in, 1 out]
                  }
                }
              }
              frame #1 {
                n978 = disable-structure shown="禁用" {
                  frame Disabled {
                    n979 = flat-sequence {
                      tunnel: [w1453] -> w1448
                      tunnel: w1448 -> [w1455]
                      tunnel: [w1455] -> w1447
                      tunnel: w1447 -> [w1456]
                      tunnel: [w1456] -> w1446
                      tunnel: w1446 -> [w1465]
                      tunnel: [w1464] -> w1445
                      tunnel: w1445 -> [w1467]
                      tunnel: [w1467] -> w1444
                      tunnel: w1444 -> [w1469]
                      tunnel: [w1468] -> w1443
                      tunnel: w1443 -> [w1478]
                      tunnel: [w1478] -> w1442
                      tunnel: w1442 -> [w1486]
                      frame #0 {
                        n980 = local write "旋转齿条轴速度(°/s)"(5.0 ("电动缸速度(mm/s)")) -> ()
                      }
                      frame #1 {
                        n981 = local read "旋转齿条电机"() -> (w1450:u32)
                        n982 = call <userlib>:"Acm_AxHome.vi"("DirMode"=u32 0, "HomeMode"=u32 11, "AxisHandle"=w1450) -> ("AxisHandle"=w1453:u32)  [unwired: 1 in, 2 out]
                      }
                      frame #2 {
                        n983 = Wait Until Next ms Multiple(millisecond multiple=u32 100 ("毫秒倍数")) -> ()  [unwired: 1 out]
                      }
                      frame #3 {
                        n984 = while {
                          tunnel: w1456 -> [w1463]
                          stop <- w1457 stop-if-true
                          n985 = call <userlib>:"Acm_AxGetCmdVelocity.vi"("AxisHandle"=w1463) -> ("Velocity"=w1462:dbl)  [unwired: 1 in, 3 out]
                          n986 = Wait Until Next ms Multiple(millisecond multiple=u32 50 ("毫秒倍数")) -> ()  [unwired: 1 out]
                          n987 = Equal To 0?(x=w1462) -> (x = 0?=w1458:bool)
                          n988 = local read "急停"() -> (w1460:bool)
                          n989 = local read "复位"() -> (w1459:bool)
                          n990 = Compound Arithmetic op=OR(invert w1460, w1459, w1458) -> (w1457:bool)
                        }
                      }
                      frame #4 {
                        n991 = call "PCI1220U角度置零.vi"("AxisHandle IN"=w1465) -> ("AxisHandle OUT"=w1464:u32)  [unwired: 10 in]
                      }
                      frame #5 {
                        n992 = Wait (ms)(milliseconds to wait=u32 100 ("等待时间（毫秒）")) -> ()  [unwired: 1 out]
                      }
                      frame #6 {
                        n993 = while {
                          tunnel: [w1476] -> w1468
                          tunnel: w1469 -> [w1474]
                          stop <- w1471 stop-if-true
                          n994 = call "PCI1220U扭矩轴位置模式.vi"("Distance"=10.0, "AxisHandle IN"=w1474) -> ("AbsSuccess"=w1470:bool, "AxisHandle OUT"=w1476:u32)  [unwired: 8 in]
                          n995 = Wait Until Next ms Multiple(millisecond multiple=u32 50 ("毫秒倍数")) -> ()  [unwired: 1 out]
                          n996 = local read "急停"() -> (w1473:bool)
                          n997 = local read "复位"() -> (w1472:bool)
                          n998 = Compound Arithmetic op=OR(invert w1473, w1472, w1470) -> (w1471:bool)
                        }
                      }
                      frame #7 {
                        n999 = while {
                          tunnel: w1478 -> [w1484]
                          stop <- w1479 stop-if-true
                          n1000 = call <userlib>:"Acm_AxGetCmdVelocity.vi"("AxisHandle"=w1484) -> ("Velocity"=w1485:dbl)  [unwired: 1 in, 3 out]
                          n1001 = Wait Until Next ms Multiple(millisecond multiple=u32 50 ("毫秒倍数")) -> ()  [unwired: 1 out]
                          n1002 = Equal To 0?(x=w1485) -> (x = 0?=w1480:bool)
                          n1003 = local read "急停"() -> (w1482:bool)
                          n1004 = local read "复位"() -> (w1481:bool)
                          n1005 = Compound Arithmetic op=OR(w1480, invert w1482, w1481) -> (w1479:bool)
                        }
                      }
                      frame #8 {
                        n1006 = call "PCI1220U角度置零.vi"("AxisHandle IN"=w1486) -> ()  [unwired: 10 in, 1 out]
                      }
                    }
                  }
                  frame Enabled {
                  }
                }
              }
              frame #2 {
                n1007 = flat-sequence {
                  frame #0 {
                    n1008 = while {
                      stop <- w1487 stop-if-true
                      n1009 = local read "电动缸回零"() -> (w1494:bool)
                      n1010 = local write "回零完成"(TRUE ("回零完成")) -> ()
                      n1011 = local write "电动缸回零"(FALSE ("电动缸回零")) -> ()
                      n1012 = Wait Until Next ms Multiple(millisecond multiple=u32 50 ("毫秒倍数")) -> ()  [unwired: 1 out]
                      n1013 = Not(x=w1494) -> (.not. x?=w1488:bool)
                      n1014 = local read "急停"() -> (w1489:bool)
                      n1015 = local read "复位"() -> (w1490:bool)
                      n1016 = Compound Arithmetic op=OR(w1488, invert w1489, w1490) -> (w1487:bool)
                    }
                  }
                }
              }
            }
          }
        }
      }
    }
    n1017 = Wait (ms)(milliseconds to wait=u32 50 ("毫秒倍数")) -> ()  [unwired: 1 out]
    n1018 = local read "停止"() -> (w1190:bool)
  }
  n1019 = while {
    stop <- FALSE stop-if-true
    n1020 = Equal?(x="密码", y="jizhuan") -> (x = y?=w1498:bool)
    n1021 = Compound Arithmetic op=AND(w1498, "?") -> (w1496:bool)
    n1022 = case shown="假" w1496 {
      frame False {
        n1023 = property class="Bool (严格)"("DisabledEnum"=T5."Disabled and Grayed Out" ("禁用")) -> ()  [unwired: 2 in, 2 out]
        n1024 = property class="Bool (严格)"("DisabledEnum"=T5."Disabled and Grayed Out" ("禁用")) -> ()  [unwired: 2 in, 2 out]
      }
      frame True {
        n1025 = property class="Bool (严格)"("DisabledEnum"=T5."Enabled" ("禁用")) -> ()  [unwired: 2 in, 2 out]
        n1026 = property class="Bool (严格)"("DisabledEnum"=T5."Enabled" ("禁用")) -> ()  [unwired: 2 in, 2 out]
        n1027 = case shown="真" "?" {
          frame False {
          }
          frame True {
            n1028 = property on="选项卡控件" class="TabCtl (严格)"() -> ("Pages"=w1507:refnum<vi>[])  [unwired: 2 in, 2 out]
            n1029 = for {
              N: 7 -> [_]
              tunnel: w1507 -> [w1509] mode=indexing
              i -> [w1510]
              n1030 = case shown="5" w1510 {
                tunnel: w1509 -> [_ w1512]
                frame 0, Default {
                }
                frame 5 {
                  n1031 = property class="Page"(reference=w1512, "PageVis"=FALSE ("选项卡可见")) -> ()  [unwired: 1 in, 2 out]
                }
              }
            }
          }
        }
        n1032 = case shown="真" "?" {
          frame False {
          }
          frame True {
            n1033 = property on="选项卡控件" class="TabCtl (严格)"() -> ("Pages"=w1513:refnum<vi>[])  [unwired: 2 in, 2 out]
            n1034 = for {
              N: 7 -> [_]
              tunnel: w1513 -> [w1515] mode=indexing
              i -> [w1516]
              n1035 = case shown="5" w1516 {
                tunnel: w1515 -> [_ w1518]
                frame 0, Default {
                }
                frame 5 {
                  n1036 = property class="Page"(reference=w1518, "PageVis"=TRUE ("选项卡可见")) -> ()  [unwired: 1 in, 2 out]
                }
              }
            }
          }
        }
      }
    }
  }
  n1037 = flat-sequence {
    tunnel: [w1522] -> w2
    tunnel: [w1520] -> w1
    tunnel: w2 -> [w1532]
    tunnel: w1 -> [w1531]
    frame #0 {
      n1038 = First Call?() -> (First Call?: T/F=w1519:bool)
      n1039 = case shown="真" w1519 {
        frame False {
        }
        frame True {
          n1040 = while {
            i -> [w1528]
            stop <- w1526 stop-if-true
            w1525 = FALSE ("回零完成")
            w1530 = TRUE ("电动缸使能")
            n1041 = local write "回零完成"(w1525) -> ()
            n1042 = local write "测头机构轴使能"(w1530) -> ()
            n1043 = local write "旋转齿条轴使能"(w1525) -> ()
            n1044 = local write "电动缸使能"(w1530) -> ()
            n1045 = Wait Until Next ms Multiple(millisecond multiple=u32 50 ("毫秒倍数")) -> ()  [unwired: 1 out]
            n1046 = Greater Or Equal?(x=w1528, y=30) -> (x >= y?=w1526:bool)
          }
        }
      }
      n1047 = call "ADO Connection Create.vi"() -> ("error out"=w1523:errorcluster, "ADODB._Connection Out"=w1524:refnum<k7>)  [unwired: 10 in]
      n1048 = call "ADO Connection Open.vi"("error in (no error)"=w1523, "ConnectionString"="Provider=Microsoft.Jet.OLEDB.4.0;Data Source=D:\\Q14070-Z060人机界面\\参数\\参数Z060.mdb;Persist Security Info=False;Jet OLEDB:Database Password=1234;", "ADODB._Connection In"=w1524) -> ("error out"=w1520:errorcluster, "ADODB._Connection Out"=w1522:refnum<k7>)  [unwired: 7 in]
    }
    frame #1 {
      n1049 = while {
        tunnel: w1532 -> [w1534]
        tunnel: w1531 -> [w1533]
        stop <- w1538 stop-if-true
        n1050 = Wait (ms)(milliseconds to wait=u32 50 ("等待时间（毫秒）")) -> ()  [unwired: 1 out]
        n1051 = First Call?() -> (First Call?: T/F=w1537:bool)
        n1052 = Or(x=w1537, y="参数加载") -> (x .or. y?=w1536:bool)
        n1053 = case shown="真" w1536 {
          tunnel: w1534 -> [_ w1541]
          tunnel: w1533 -> [_ w1540]
          frame False {
          }
          frame True {
            n1054 = stacked-sequence {
              tunnel: w1541 -> [w1547 w1558 w1601]
              tunnel: w1540 -> [w1542 _ _]
              frame #0 {
                n1055 = call "SQL Execute.vi"("error in (no error)"=w1542, "Command Text"="SELECT * FROM 测试参数表", "ADODB._Connection In"=w1547) -> ("Data"=w1545:string[][])  [unwired: 5 in, 3 out]
                n1056 = Index Array(array=w1545, index (col)=0 ("索引 (行)")) -> (element=w1549:string[])  [unwired: 1 in]
                n1057 = Array Size(array=w1549) -> (size(s)=w1544:i32)
                "型号数量" <- w1544
                n1058 = while {
                  shift-right: [w1556] -> w1548
                  shift-left: i32[] [] -> [w1555]
                  tunnel: w1544 -> [w1553]
                  i -> [w1554]
                  stop <- w1552 stop-if-true
                  n1059 = Greater Or Equal?(x=w1554, y=w1553) -> (x >= y?=w1552:bool)
                  n1060 = Build Array (concatenate)(w1555, w1554) -> (w1556:i32[])
                }
                n1061 = Build Cluster Array "索引与捆绑簇数组"(w1549, w1548) -> (w1543:cluster{"String":string, i32}[])
                n1062 = property on="型号选择" class="Ring (严格)"("StringsAndValues[]"=w1543) -> ()  [unwired: 2 in, 2 out]
              }
              frame #1 {
                n1063 = property on="型号选择" class="Ring (严格)"() -> ("RingText.Text"=w1559:string)  [unwired: 2 in, 2 out]
                n1064 = call "创建文本2"("型号选择"=w1559) -> ("Result"=w1563:string)  [unwired: 13 in, 1 out]
                n1065 = call "SQL Execute.vi"("Command Text"=w1563, "ADODB._Connection In"=w1558) -> ("Data"=w1562:string[][])  [unwired: 6 in, 3 out]
                n1066 = Index Array(array=w1562, index (row)=0 ("索引 (行)")) -> (element=w1560:string[])  [unwired: 1 in]
                n1067 = Fract/Exp String To Number ("分数/指数字符串至数值转换")(string=w1560) -> (number=w1557:dbl[])  [unwired: 3 in, 1 out]
                n1068 = stacked-sequence {
                  tunnel: w1557 -> [w1586]
                  frame #0 {
                    n1069 = Index Array ("索引数组")(array=w1586, index #1=2 ("索引")) -> (element #1=w1585:dbl, element #2=w1584:dbl, element #3=w1583:dbl, element #4=w1582:dbl, element #5=w1581:dbl, element #6=w1580:dbl, element #7=w1579:dbl, element #8=w1578:dbl, element #9=w1577:dbl, element #10=w1576:dbl, element #11=w1575:dbl, element #12=w1574:dbl, element #13=→"齿条传动比":dbl, element #14=→"力波动标准(N)":dbl, element #15=→"轴向力标准(N)":dbl, element #16=→"平均轴向力标准(N) max":dbl, element #17=→"总圈数标准":dbl, element #18=→"总圈数最大值":dbl, element #19=w1573:dbl, element #20=w1566:dbl, element #21=w1565:dbl, element #22=w1564:dbl)  [unwired: 21 in]
                    n1070 = local write "测头机构轴移动速度"(w1585) -> ()
                    n1071 = local write "中间位置最大间隙标准(mm)"(w1566) -> ()
                    n1072 = local write "测头机构轴检测位"(w1584) -> ()
                    n1073 = local write "测头机构轴后退位"(w1582) -> ()
                    n1074 = local write "180°外全行程间隙标准(mm)"(w1564) -> ()
                    n1075 = local write "测头机构轴待检位"(w1583) -> ()
                    n1076 = local write "180°内全行程间隙标准(mm)"(w1565) -> ()
                    n1077 = local write "旋转齿条轴找帽转速"(w1578) -> ()
                    n1078 = local write "旋转齿条轴测量转速"(w1577) -> ()
                    n1079 = local write "转向器中心"(w1573) -> ()
                    n1080 = local write "总行程标准(mm)"(w1575) -> ()
                    n1081 = local write "齿条移动速度"(w1581) -> ()
                    n1082 = local write "齿条左极限"(w1580) -> ()
                    n1083 = local write "齿条右极限"(w1579) -> ()
                    n1084 = local write "总行程最大值"(w1574) -> ()
                    n1085 = local write "测量点扭矩"(w1576) -> ()
                  }
                }
              }
              frame #2 {
                n1086 = call "SQL Execute.vi"("Command Text"="SELECT * FROM 传感器校验表 where ID='1'", "ADODB._Connection In"=w1601) -> ("Data"=w1603:string[][])  [unwired: 6 in, 3 out]
                n1087 = Index Array(array=w1603) -> (element=w1604:string[])  [unwired: 2 in]
                n1088 = Fract/Exp String To Number ("分数/指数字符串至数值转换")(string=w1604) -> (number=w1594:dbl[])  [unwired: 3 in, 1 out]
                n1089 = Index Array(array=w1594, index #1=1 ("索引"), index #2=2 ("索引"), index #3=3 ("索引"), index #4=4 ("索引"), index #5=5 ("索引"), index #6=6 ("索引")) -> (element #1=w1593:dbl, element #2=w1592:dbl, element #3=w1591:dbl, element #4=w1590:dbl, element #5=w1589:dbl, element #6=w1588:dbl)
                n1090 = local write "间隙位移零点偏移"(w1593) -> ()
                n1091 = local write "间隙位移比例偏移"(w1592) -> ()
                n1092 = local write "齿条推拉力零点偏移"(w1591) -> ()
                n1093 = local write "齿条推拉力比例偏移"(w1590) -> ()
                n1094 = local write "齿条扭矩零点偏移"(w1589) -> ()
                n1095 = local write "齿条扭矩比例偏移"(w1588) -> ()
              }
            }
          }
        }
        n1096 = local read "停止"() -> (w1538:bool)
        "ADODB._Connection Out 2" <- w1534
      }
    }
  }
  n1097 = while {
    stop <- w1606 stop-if-true
    n1098 = local read "rfid工步号"() -> (w1605:u32)
    n1099 = case shown="10" w1605 {
      frame 0, Default {
      }
      frame 10 {
        n1100 = flat-sequence {
          tunnel: [w1616] -> w1610
          tunnel: w1610 -> [w1618]
          tunnel: [w1617] -> w1609
          tunnel: w1609 -> [w1620]
          tunnel: [w1620] -> w1608
          tunnel: w1608 -> [w1623]
          frame #0 {
            n1101 = while {
              stop <- w1611 stop-if-true
              n1102 = local read "rfid触发"() -> (w1611:bool)
              n1103 = Wait Until Next ms Multiple(millisecond multiple=u32 50 ("毫秒倍数")) -> ()  [unwired: 1 out]
            }
          }
          frame #1 {
            n1104 = local write "芯片ID"("" ("随行板ID")) -> ()
            n1105 = local write "rfid完成"(FALSE ("RFID完成")) -> ()
            n1106 = local write "rfid触发"(FALSE ("RFID读取触发")) -> ()
          }
          frame #2 {
            n1107 = local read "Z060BRFID"() -> (w1616:string)
            n1108 = local write "芯片ID"(w1616) -> ()
          }
          frame #3 {
            n1109 = call "查询产品ID.vi"("芯片编码"=w1618) -> ("产品ID"=w1617:string)  [unwired: 8 in, 2 out]
            "读取产品ID" <- w1617
          }
          frame #4 {
            n1110 = Wait (ms)(milliseconds to wait=u32 500 ("等待时间（毫秒）")) -> ()  [unwired: 1 out]
          }
          frame #5 {
            n1111 = call "查询上序合格.vi"("产品ID"=w1623) -> ("本序已做"=w1621:bool, "上序合格"=w1622:bool)  [unwired: 8 in, 1 out]
            n1112 = Not(x=w1622) -> (.not. x?=w1624:bool)
            n1113 = local write "上序合格"(w1622) -> ()
            n1114 = local write "本序已做"(w1621) -> ()
            n1115 = local write "上序不合格"(w1624) -> ()
          }
          frame #6 {
            n1116 = local write "rfid完成"(TRUE ("RFID读取完成")) -> ()
            n1117 = Wait Until Next ms Multiple(millisecond multiple=u32 500 ("毫秒倍数")) -> ()  [unwired: 1 out]
          }
          frame #7 {
            "rfid工步号" <- 15.0 ("工步号")
          }
        }
      }
      frame 210 {
        n1118 = local read "读取产品ID"() -> (w1628:string)
        n1119 = local write "产品ID"(w1628) -> ()
      }
    }
    n1120 = Wait Until Next ms Multiple(millisecond multiple=u32 50 ("毫秒倍数")) -> ()  [unwired: 1 out]
    n1121 = local read "停止"() -> (w1606:bool)
  }
  n1122 = flat-sequence {
    tunnel: [w1629] -> w4
    tunnel: w4 -> [w1635]
    tunnel: [w1634] -> w3
    tunnel: w3 -> [w1705]
    frame #0 {
      n1123 = call "PCI1240U初始化.vi"() -> ("旋转电机"=→"旋转齿条电机":u32, "电动缸电机"=→"电动缸电机":u32, "DeviceHandle"=→"DeviceHandle":u32, "进给电机"=→"测头机构电机":u32)  [unwired: 6 in, 2 out]
      n1124 = call "PCI8622配置.vi"() -> ("DeviceID"=w1629:i32)  [unwired: 11 in]
    }
    frame #1 {
      n1125 = while {
        tunnel: w1635 -> [w1637]
        tunnel: [w1636] -> w1634
        stop <- "停止" stop-if-true
        n1126 = stacked-sequence {
          tunnel: w1637 -> [_ _ w1681]
          tunnel: [_ _ w1681] -> w1636
          frame #0 {
            n1127 = local read "测头机构电机"() -> (w1646:u32)
            n1128 = Boolean To (0,1)(Boolean="测头机构轴使能") -> (0, 1=w1644:i16)
            n1129 = call <userlib>:"Acm_AxSetSvOn.vi"("OnOff"=w1644, "AxisHandle"=w1646) -> ("AxisHandle"=w1643:u32)  [unwired: 1 in, 2 out]
            n1130 = call "PCI1220U进给轴速度设置.vi"("Change Velocity"="测头机构轴速度(mm/s)", "AxisHandle IN"=w1643) -> ("AxisHandle OUT"=w1641:u32)  [unwired: 9 in]
            n1131 = call "PCI1220U进给轴读取位置.vi"("AxisHandle IN"=w1641) -> ("位置"=→"测头机构轴位置(mm)":dbl)  [unwired: 9 in, 1 out]
          }
          frame #1 {
            n1132 = local read "电动缸电机"() -> (w1656:u32)
            n1133 = local read "旋转齿条电机"() -> (w1655:u32)
            n1134 = Boolean To (0,1)(Boolean="电动缸使能") -> (0, 1=w1660:i16)
            n1135 = Boolean To (0,1)(Boolean="旋转齿条轴使能") -> (0, 1=w1654:i16)
            n1136 = call <userlib>:"Acm_AxSetSvOn.vi"("OnOff"=w1654, "AxisHandle"=w1655) -> ("AxisHandle"=w1657:u32)  [unwired: 1 in, 2 out]
            n1137 = call <userlib>:"Acm_AxSetSvOn.vi"("OnOff"=w1660, "AxisHandle"=w1656) -> ("AxisHandle"=w1659:u32)  [unwired: 1 in, 2 out]
            n1138 = call "PCI1220U扭矩轴速度设置.vi"("Change Velocity"="旋转齿条轴速度(°/s)", "AxisHandle IN"=w1657) -> ("AxisHandle OUT"=w1658:u32)  [unwired: 9 in]
            n1139 = call "PCI1240电动缸速度设置.vi"("Change Velocity"="电动缸速度(mm/s)", "AxisHandle IN"=w1659) -> ("AxisHandle OUT"=w1647:u32)  [unwired: 9 in]
            n1140 = call "PCI1220U扭矩轴读取位置.vi"("AxisHandle IN"=w1658) -> ("位置"=→"旋转齿条轴位置(°)":dbl)  [unwired: 9 in, 1 out]
            n1141 = call "PCI1240电动缸读取位置.vi"("AxisHandle IN"=w1647) -> ("位置"=→"电动缸位置(mm)":dbl)  [unwired: 9 in, 1 out]
          }
          frame #2 {
            w1697 = 0  # nRetSizeWords
            w1698 = 2048  # nReadSizeWords
            # "hDevice"
            n1142 = Initialize Array(u16 0, 2048 ("dimension size")) -> (w1688:u16[])
            n1143 = dll-call lib="PCI8622_32.dll" fn="PCI8622_ReadDeviceProAD_Npt" label="ReadDeviceProAD_Npt"("hDevice"=w1681, "ADBuffer[]"=w1688, "nReadSizeWords"=w1698, "nRetSizeWords"=w1697) -> ("ADBuffer[]"=w1691:u16[])  [unwired: 7 in, 2 out]
            n1144 = Divide(x=w1691, y=65536.01) -> (x/y=w1692:dbl[])
            n1145 = Multiply(x=w1692, y=20) -> (x*y=w1695:dbl[])
            n1146 = Subtract(x=w1695, y=10) -> (x-y=w1687:dbl[])
            n1147 = Decimate 1D Array ("抽取一维数组")(w1687) -> (w1675:dbl[], w1676:dbl[], w1674:dbl[])  [unwired: 5 out]
            n1148 = Add Array Elements(numeric array=w1674) -> (sum=w1685:dbl)
            n1149 = Array Size(array=w1674) -> (size(s)=w1686:i32)
            n1150 = Divide(x=w1685, y=w1686) -> (x/y=w1667:dbl)
            n1151 = Divide(x=w1667, y=5.86) -> (x/y=w1664:dbl)
            n1152 = Multiply(x=4.0, y=w1664) -> (x*y=w1662:dbl)
            n1153 = Add Array Elements(numeric array=w1675) -> (sum=w1684:dbl)
            n1154 = Array Size(array=w1675) -> (size(s)=w1683:i32)
            n1155 = Add Array Elements(numeric array=w1676) -> (sum=w1680:dbl)
            n1156 = Array Size(array=w1676) -> (size(s)=w1682:i32)
            n1157 = Divide(x=w1684, y=w1683) -> (x/y=w1673:dbl)
            n1158 = Divide(x=w1680, y=w1682) -> (x/y=w1670:dbl)
            n1159 = Multiply(x=w1673, y=2.0) -> (x*y=w1668:dbl)
            n1160 = Multiply(x=w1670, y=200.0) -> (x*y=w1669:dbl)
            n1161 = Subtract(x=w1662, y=0.675) -> (x-y=w1665:dbl)
            n1162 = local read "间隙位移比例偏移"() -> (w1702:dbl)
            n1163 = local read "间隙位移零点偏移"() -> (w1701:dbl)
            n1164 = local read "齿条扭矩零点偏移"() -> (w1703:dbl)
            n1165 = local read "齿条扭矩比例偏移"() -> (w1704:dbl)
            n1166 = local read "齿条推拉力比例偏移"() -> (w1700:dbl)
            n1167 = local read "齿条推拉力零点偏移"() -> (w1699:dbl)
            n1168 = call "传感器校订.vi"("零点"=w1703, "比例"=w1704, "传感器"=w1668) -> ("示值"=→"齿条扭矩(Nm)":dbl)  [unwired: 8 in]
            n1169 = call "传感器校订.vi"("零点"=w1701, "比例"=w1702, "传感器"=w1665) -> ("示值"=→"间隙位移(mm)":dbl)  [unwired: 8 in]
            n1170 = call "传感器校订.vi"("零点"=w1699, "比例"=w1700, "传感器"=w1669) -> ("示值"=→"齿条推拉力(N)":dbl)  [unwired: 8 in]
          }
        }
        n1171 = Wait Until Next ms Multiple(millisecond multiple=u32 50 ("毫秒倍数")) -> ()  [unwired: 1 out]
      }
    }
    frame #2 {
      n1172 = dll-call lib="PCI8622_32.dll" fn="PCI8622_StopDeviceProAD" label="StopDeviceProAD"("hDevice"=w1705) -> ("hDevice"=w1706:i32)  [unwired: 4 in, 2 out]
      n1173 = dll-call lib="PCI8622_32.dll" fn="PCI8622_ReleaseDeviceProAD" label="ReleaseDeviceProAD"("hDevice"=w1706) -> ()  [unwired: 5 in, 2 out]
      n1174 = dll-call lib="PCI8622_32.dll" fn="PCI8622_ReleaseDevice" label="ReleaseDevice"("hDevice"=w1705) -> ()  [unwired: 5 in, 2 out]
    }
  }
